vi "03 Channel Tester.vi"() -> ()   [LabVIEW 2009]
uses:
  EquipReferences.ctl
  HEWH Tank Indicator.ctl
  Sensor.ctl
  <vilib>/Instr/_visa.llb/VISA Configure Serial Port (Instr).vi
  <vilib>/Analysis/NI_AALBase.lvlib
panel:
  out "Serial Loopback":cluster{"Com OK":dbl, "Color Box":u32}={"Com OK"=0.0, "Color Box"=8585007}
  in  "RTD Min OK":dbl=30.0
  in  "RTD Max OK":dbl=180.0
  in  "PSI Min OK":dbl=100.0
  in  "PSI Max OK":dbl=400.0
  in  "StDev Thresh":dbl=0.2
  in  "TC Min OK Val":dbl=20.0
  in  "TC Max OK Val":dbl=400.0
  out "Pressures":T1[](array[typedef])=[{"Mean"=0.0, " St Dev."=0.0, "Color Box"=8585007}, {"Mean"=0.0, " St Dev."=0.0, "Color Box"=8585007}, {"Mean"=0.0, " St Dev."=0.0, "Color Box"=8585007}]
  out "Temperatures":T1[](array[typedef])=[{"Mean"=0.0, " St Dev."=0.0, "Color Box"=8585007}, {"Mean"=0.0, " St Dev."=0.0, "Color Box"=8585007}, {"Mean"=0.0, " St Dev."=0.0, "Color Box"=8585007}]
  out "Tc Down":T1={"Mean"=0.0, " St Dev."=0.0, "Color Box"=8585007}
  out "Power":T1={"Mean"=0.0, " St Dev."=0.0, "Color Box"=8585007}
  in  "Panel 3":T1[][](array[typedef])=[[{"Mean"=0.0, " St Dev."=0.0, "Color Box"=8585007}, {"Mean"=0.0, " St Dev."=0.0, "Color Box"=8585007}, {"Mean"=0.0, " St Dev."=0.0, "Color Box"=8585007}, {"Mean"=0.0, " St Dev."=0.0, "Color Box"=8585007}, {"Mean"=0.0, " St Dev."=0.0, "Color Box"=8585007}, {"Mean"=0.0, " St Dev."=0.0, "Color Box"=8585007}], [{"Mean"=0.0, " St Dev."=0.0, "Color Box"=8585007}, {"Mean"=0.0, " St Dev."=0.0, "Color Box"=8585007}, {"Mean"=0.0, " St Dev."=0.0, "Color Box"=8585007}, {"Mean"=0.0, " St Dev."=0.0, "Color Box"=8585007}, {"Mean"=0.0, " St Dev."=0.0, "Color Box"=8585007}, {"Mean"=0.0, " St Dev."=0.0, "Color Box"=8585007}], [{"Mean"=0.0, " St Dev."=0.0, "Color Box"=8585007}, {"Mean"=0.0, " St Dev."=0.0, "Color Box"=8585007}, {"Mean"=0.0, " St Dev."=0.0, "Color Box"=8585007}, {"Mean"=0.0, " St Dev."=0.0, "Color Box"=8585007}, {"Mean"=0.0, " St Dev."=0.0, "Color Box"=8585007}, {"Mean"=0.0, " St Dev."=0.0, "Color Box"=8585007}]]
  in  "Panel 2":T1[][](array[typedef])=[[{"Mean"=0.0, " St Dev."=0.0, "Color Box"=8585007}, {"Mean"=0.0, " St Dev."=0.0, "Color Box"=8585007}, {"Mean"=0.0, " St Dev."=0.0, "Color Box"=8585007}, {"Mean"=0.0, " St Dev."=0.0, "Color Box"=8585007}, {"Mean"=0.0, " St Dev."=0.0, "Color Box"=8585007}, {"Mean"=0.0, " St Dev."=0.0, "Color Box"=8585007}], [{"Mean"=0.0, " St Dev."=0.0, "Color Box"=8585007}, {"Mean"=0.0, " St Dev."=0.0, "Color Box"=8585007}, {"Mean"=0.0, " St Dev."=0.0, "Color Box"=8585007}, {"Mean"=0.0, " St Dev."=0.0, "Color Box"=8585007}, {"Mean"=0.0, " St Dev."=0.0, "Color Box"=8585007}, {"Mean"=0.0, " St Dev."=0.0, "Color Box"=8585007}], [{"Mean"=0.0, " St Dev."=0.0, "Color Box"=8585007}, {"Mean"=0.0, " St Dev."=0.0, "Color Box"=8585007}, {"Mean"=0.0, " St Dev."=0.0, "Color Box"=8585007}, {"Mean"=0.0, " St Dev."=0.0, "Color Box"=8585007}, {"Mean"=0.0, " St Dev."=0.0, "Color Box"=8585007}, {"Mean"=0.0, " St Dev."=0.0, "Color Box"=8585007}]]
  in  "Panel 1":T1[][](array[typedef])=[[{"Mean"=0.0, " St Dev."=0.0, "Color Box"=8585007}, {"Mean"=0.0, " St Dev."=0.0, "Color Box"=8585007}, {"Mean"=0.0, " St Dev."=0.0, "Color Box"=8585007}, {"Mean"=0.0, " St Dev."=0.0, "Color Box"=8585007}, {"Mean"=0.0, " St Dev."=0.0, "Color Box"=8585007}, {"Mean"=0.0, " St Dev."=0.0, "Color Box"=8585007}], [{"Mean"=0.0, " St Dev."=0.0, "Color Box"=8585007}, {"Mean"=0.0, " St Dev."=0.0, "Color Box"=8585007}, {"Mean"=0.0, " St Dev."=0.0, "Color Box"=8585007}, {"Mean"=0.0, " St Dev."=0.0, "Color Box"=8585007}, {"Mean"=0.0, " St Dev."=0.0, "Color Box"=8585007}, {"Mean"=0.0, " St Dev."=0.0, "Color Box"=8585007}], [{"Mean"=0.0, " St Dev."=0.0, "Color Box"=8585007}, {"Mean"=0.0, " St Dev."=0.0, "Color Box"=8585007}, {"Mean"=0.0, " St Dev."=0.0, "Color Box"=8585007}, {"Mean"=0.0, " St Dev."=0.0, "Color Box"=8585007}, {"Mean"=0.0, " St Dev."=0.0, "Color Box"=8585007}, {"Mean"=0.0, " St Dev."=0.0, "Color Box"=8585007}]]
  out "Data Sample":i32
  out "serial error out":errorcluster
  out "Com Port Timeout Value":u32
  out "Local Tank Display":T2 {"TC6" format="%.2g"; "TIN" format="%.2g"; "TOUT" format="%.2g"; "Mean" format="%.2f"; "Std Dev" format="%.2f"; "TC5" format="%.2g"; "TC4" format="%.2g"; "TC3" format="%.2g"; "TC2" format="%.2g"; "TC1" format="%.2g"}
  in  "Num Samples":i32=5
  in  "COM Port":refnum<visa-resource-name>="COM3"
  in  "Semiphore":T3
  in  "error in (no error)":errorcluster
  in  "Equipment":T4={"COM Port"="COM1", "MW100"="MW100", "AG34970"="A-34972A", "Chamber"="WT500"}
  in  "Serial Test":bool
  in  "Test DAQ":bool
  in  "OK":bool
  # "HEWH Pannel Channel Tester"
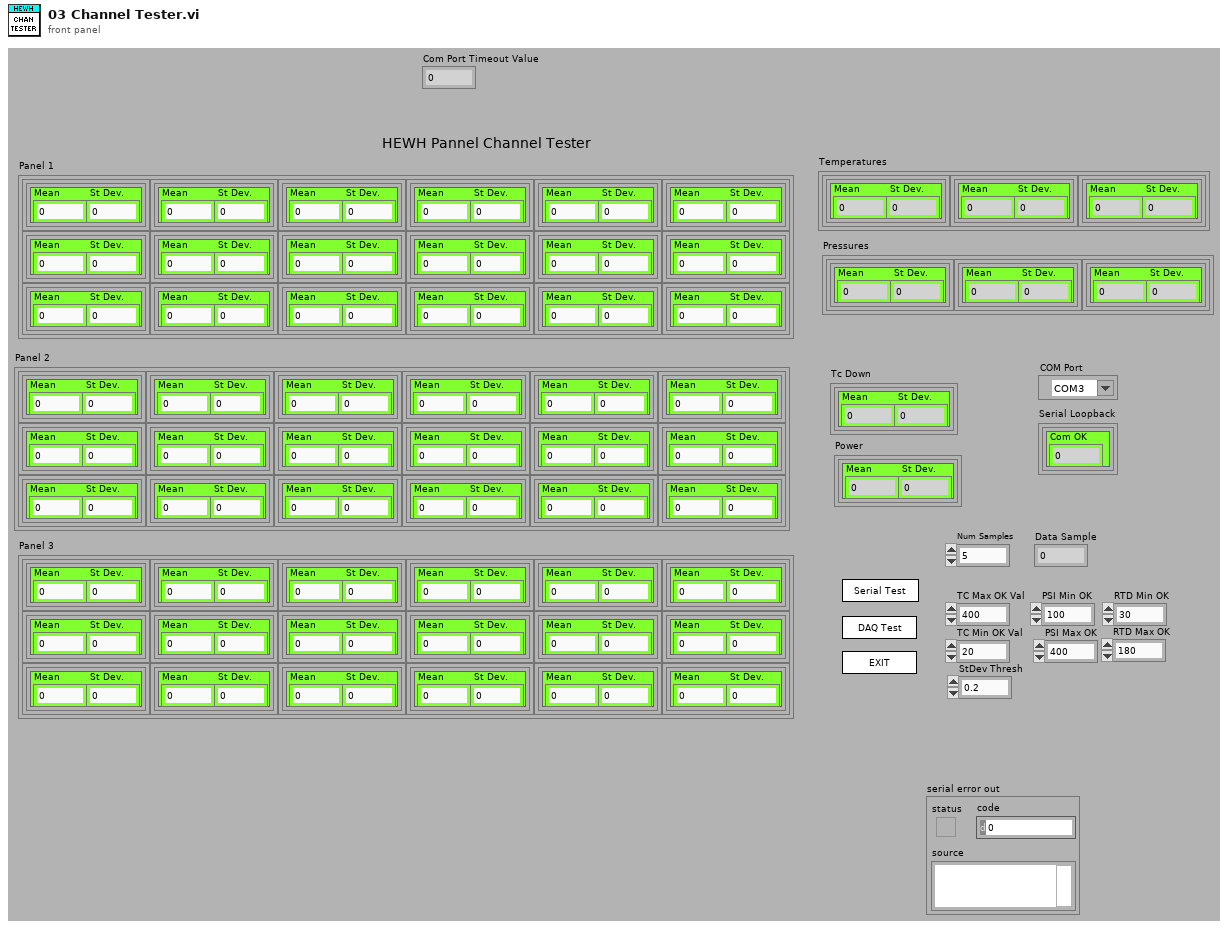
[diagram p1: front panel]
types:
  T1 = typedef "Sensor.ctl" = cluster{"Mean":dbl, " St Dev.":dbl, "Color Box":u32}
  T2 = typedef "HEWH Tank Indicator.ctl" = cluster{"TC1-D":bool, "TC2-D":bool, "TC3-D":bool, "TC4-D":bool, "TC5-D":bool, "RTD_IN":bool, "RTDOUT":bool, "TC1":dbl, "TC2":dbl, "TC3":dbl, "TC4":dbl, "TC5":dbl, "TIN":dbl, "TOUT":dbl, "Std Dev":dbl, "Mean":dbl, "TC6-D":bool, "TC6":dbl}
  T3 = typedef "Semaphore RefNum" = refnum<k1>
  T4 = typedef "EquipReferences.ctl" = cluster{"COM Port":refnum<visa-resource-name>, "MW100":refnum<visa-resource-name>, "AG34970":refnum<visa-resource-name>, "Chamber":refnum<visa-resource-name>}
  T5 = enum32{"invalid app kind", "Development System", "Run Time System", "Student Edition", "Embedded LabVIEW", "Evaluation", "Custom"}
  T6 = enum32{"Invalid", "Standard", "Closed", "Hidden", "Minimized", "Maximized"}
  T7 = cluster{"Core":cluster{"Current VI Reference":refnum<vi>, "Close Panel on Exit?":bool}, "Num Samples":i32, "Equipment Out":T4, "semaphore":T3, "Timeout":u32, "Test Data Array":T1[]}
  T8 = cluster{"Current VI Reference":refnum<vi>, "Close Panel on Exit?":bool}
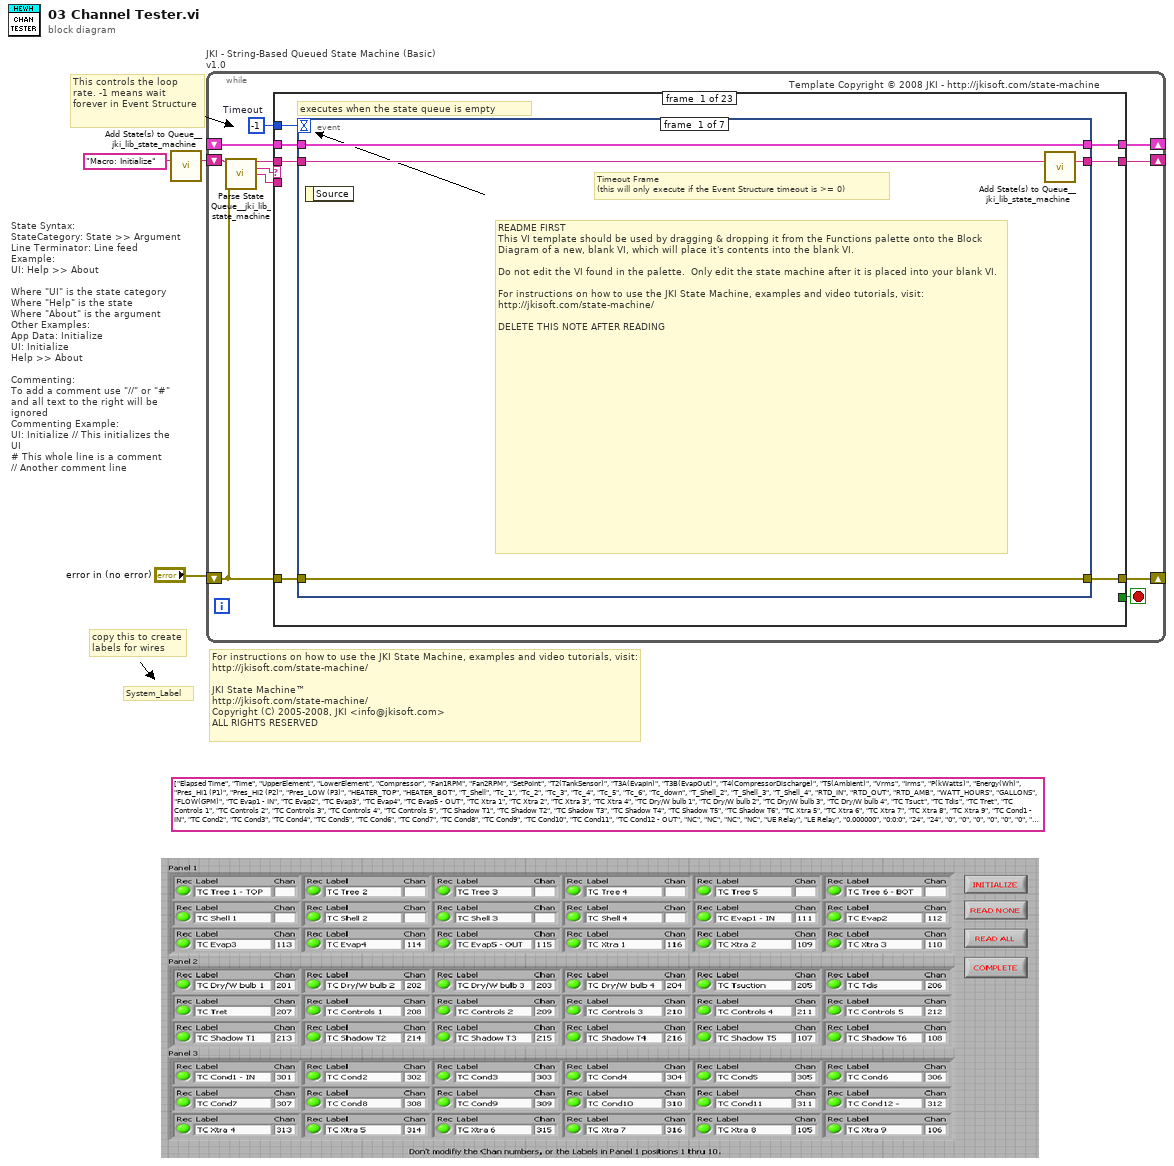
[diagram p0: block diagram]
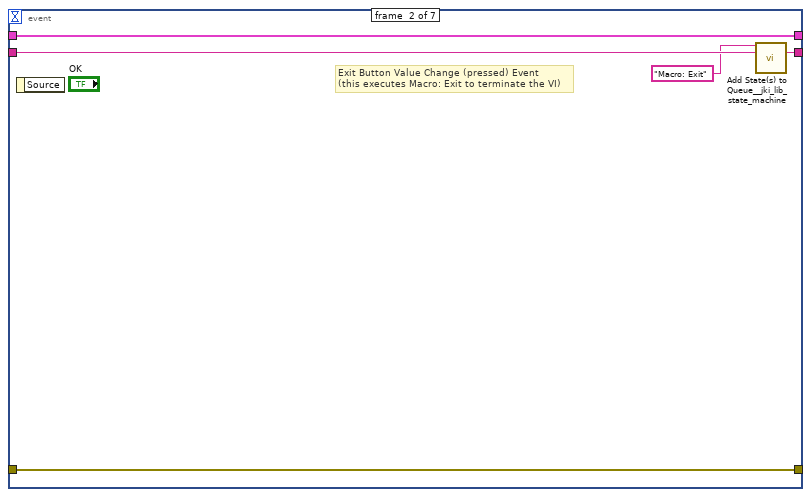
[diagram p2: hidden frame]
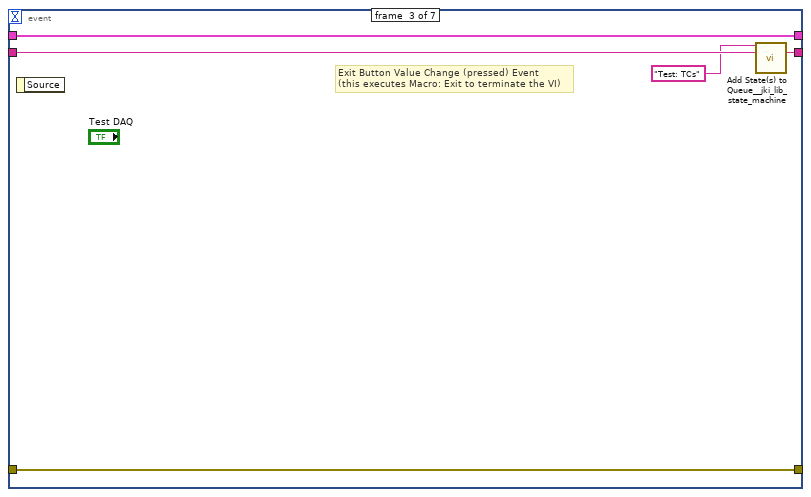
[diagram p3: hidden frame]
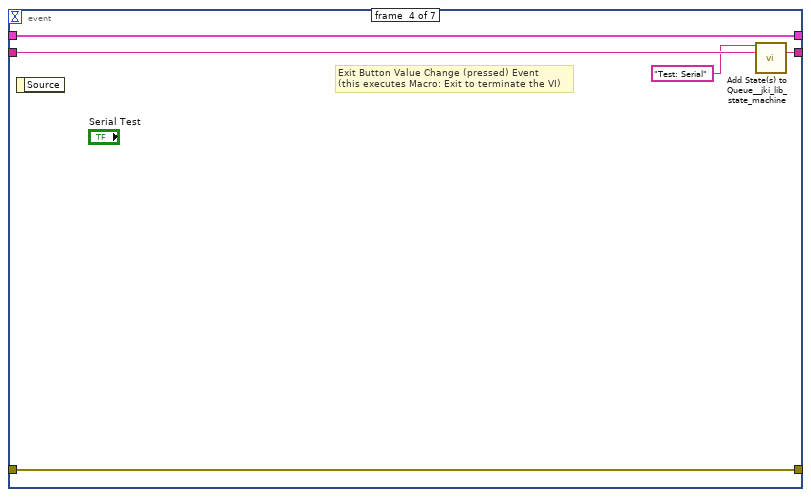
[diagram p4: hidden frame]
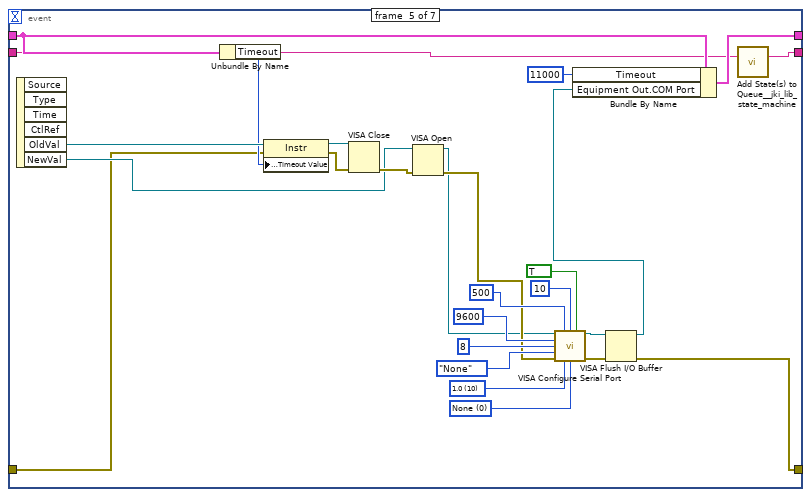
[diagram p5: hidden frame]
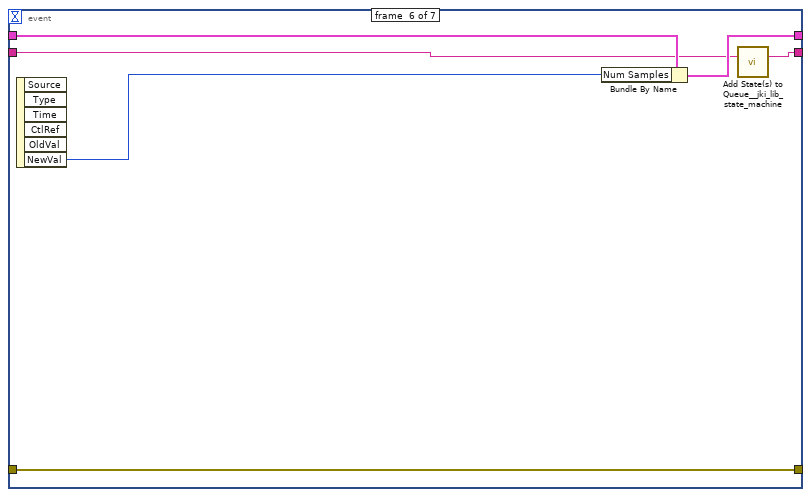
[diagram p6: hidden frame]
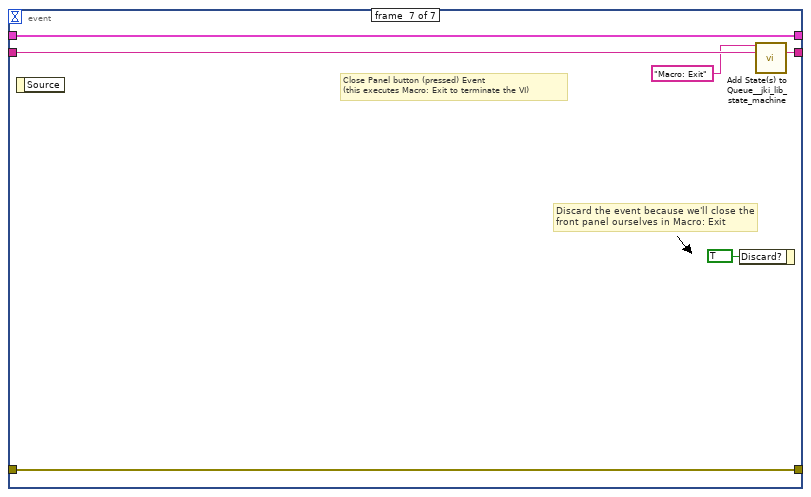
[diagram p7: hidden frame]
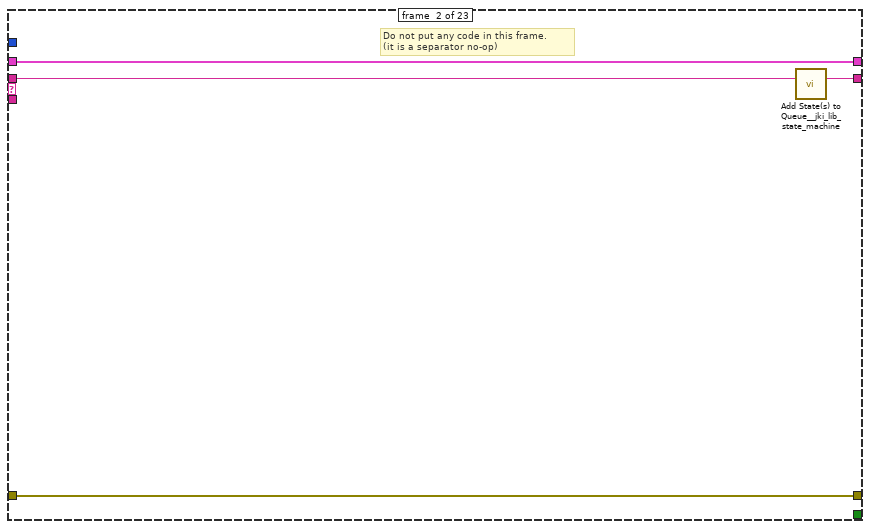
[diagram p8: hidden frame]
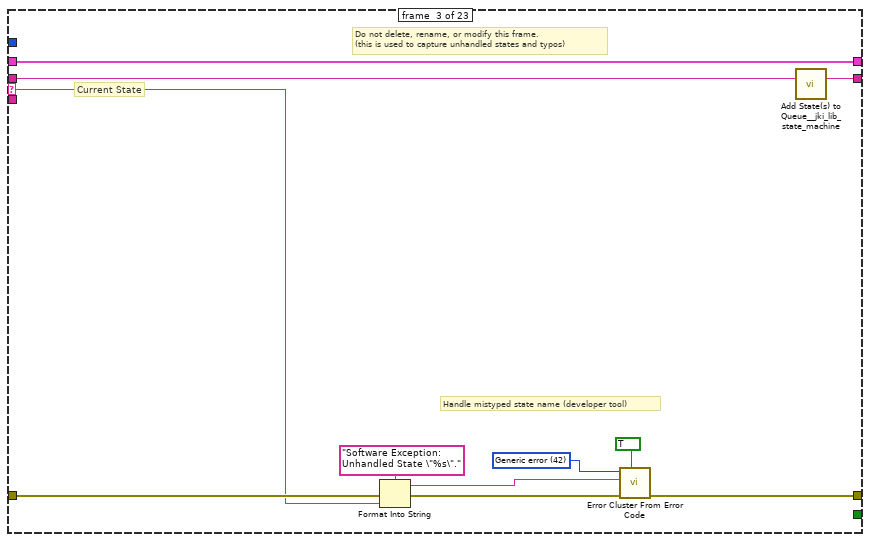
[diagram p9: hidden frame]
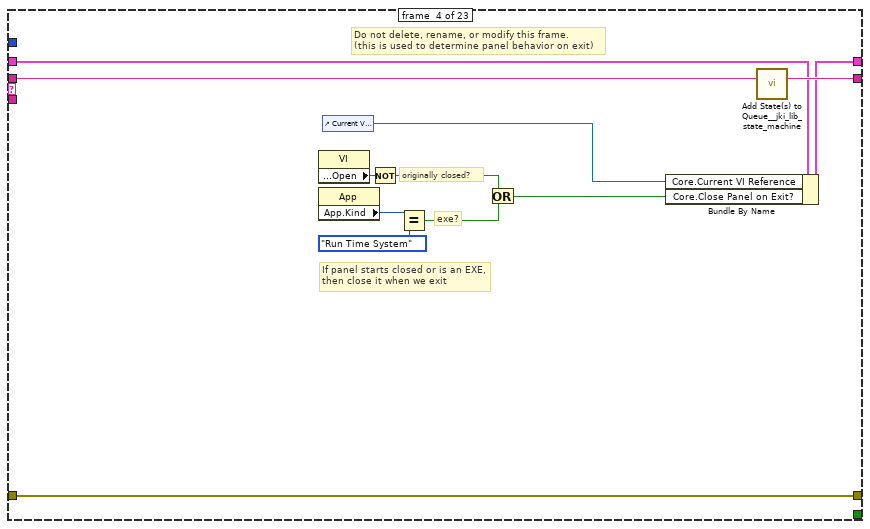
[diagram p10: hidden frame]
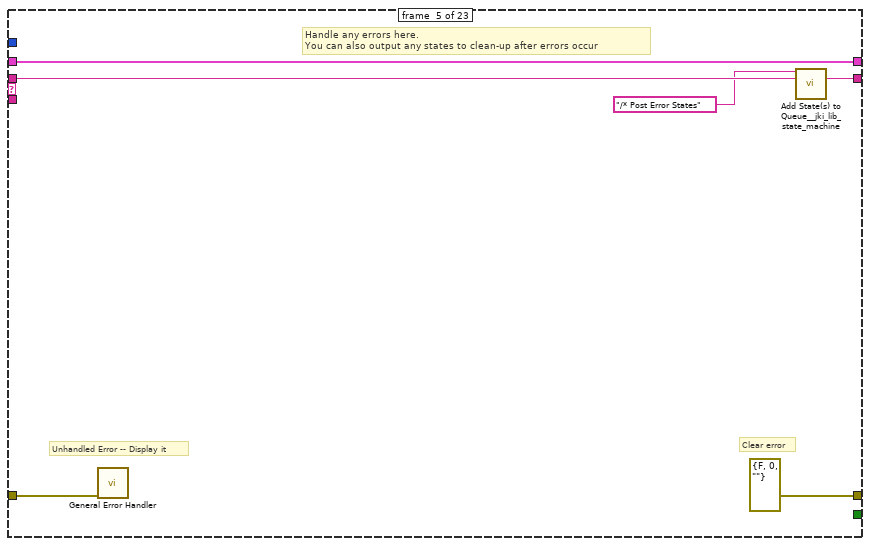
[diagram p11: hidden frame]
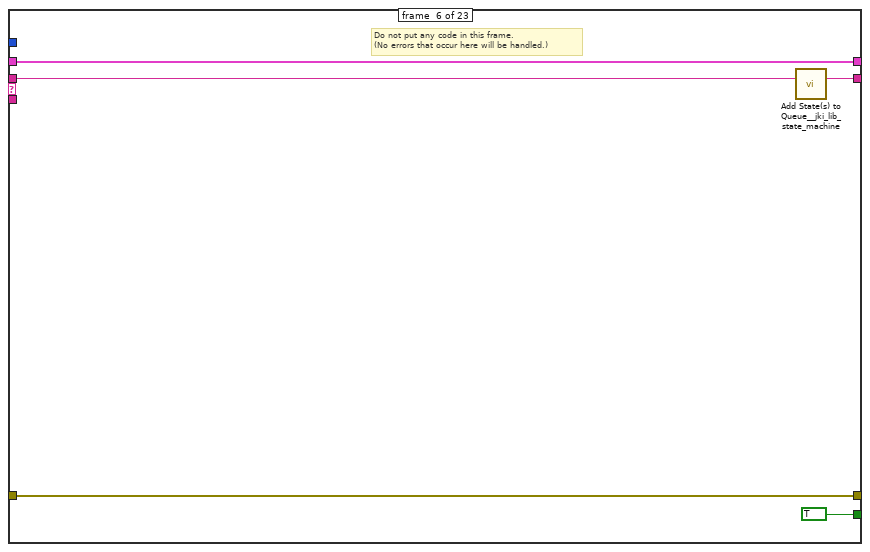
[diagram p12: hidden frame]
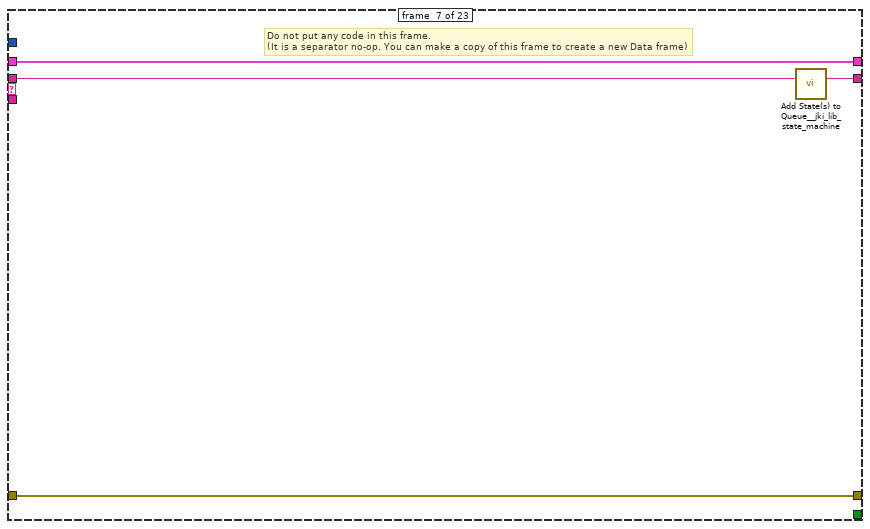
[diagram p13: hidden frame]
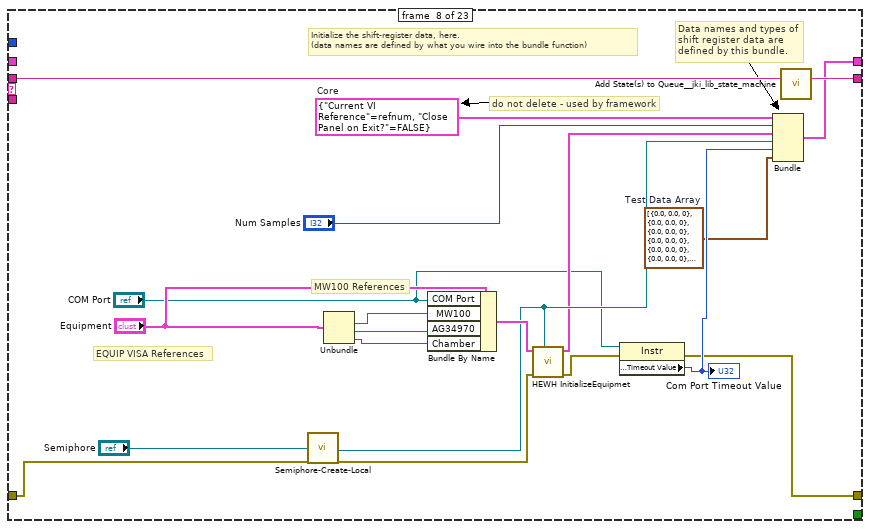
[diagram p14: hidden frame]
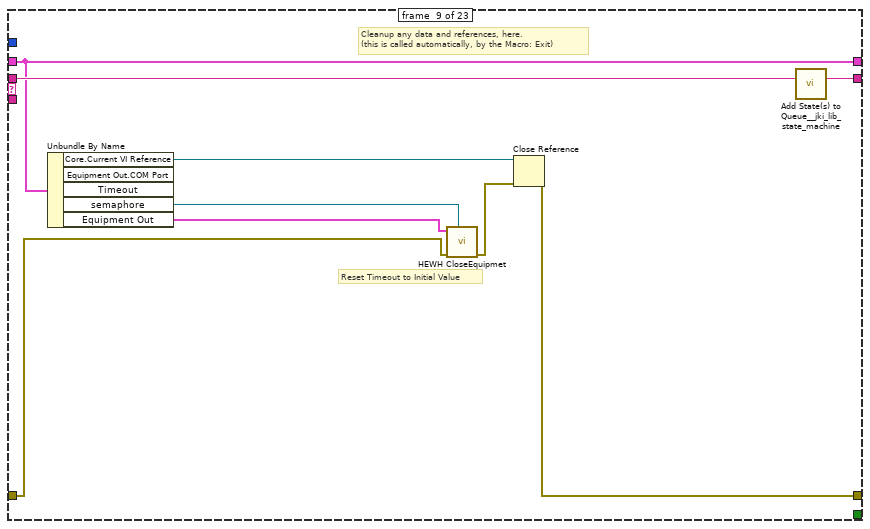
[diagram p15: hidden frame]
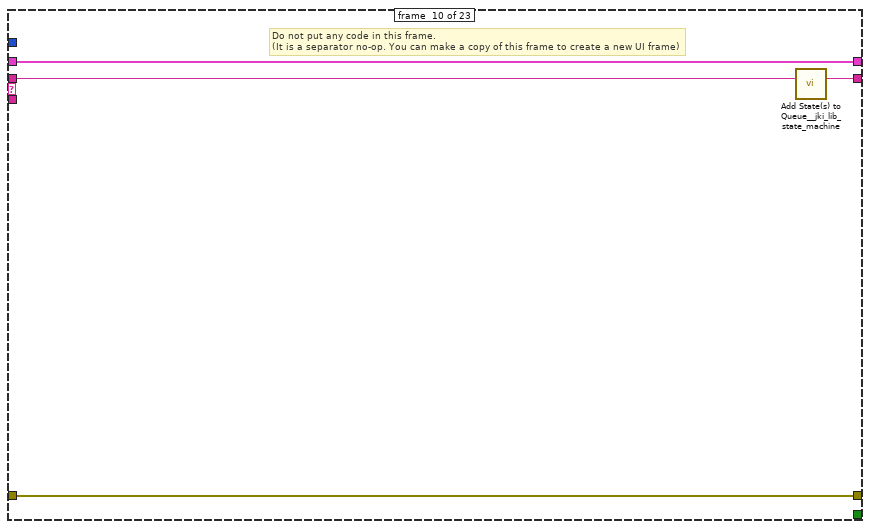
[diagram p16: hidden frame]
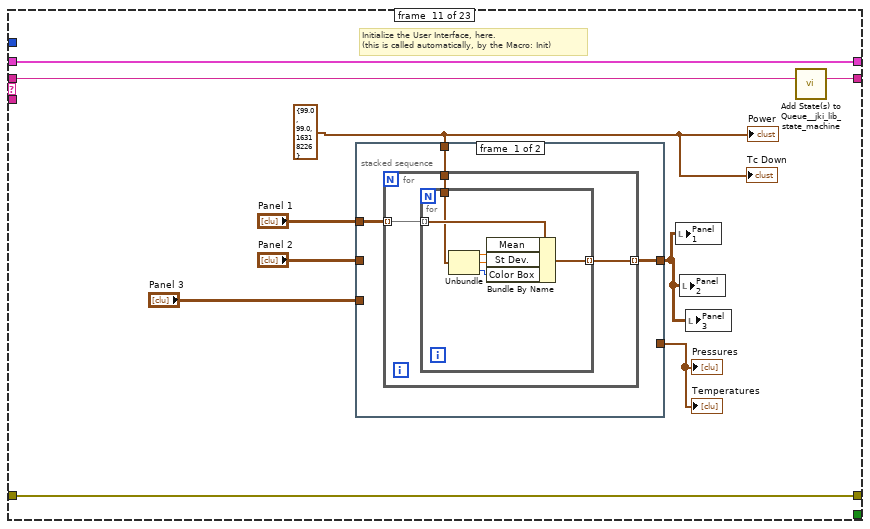
[diagram p17: hidden frame]
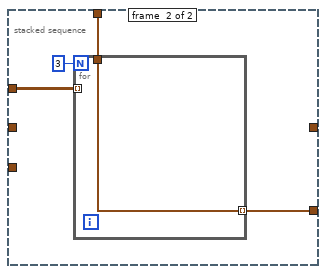
[diagram p18: hidden frame]
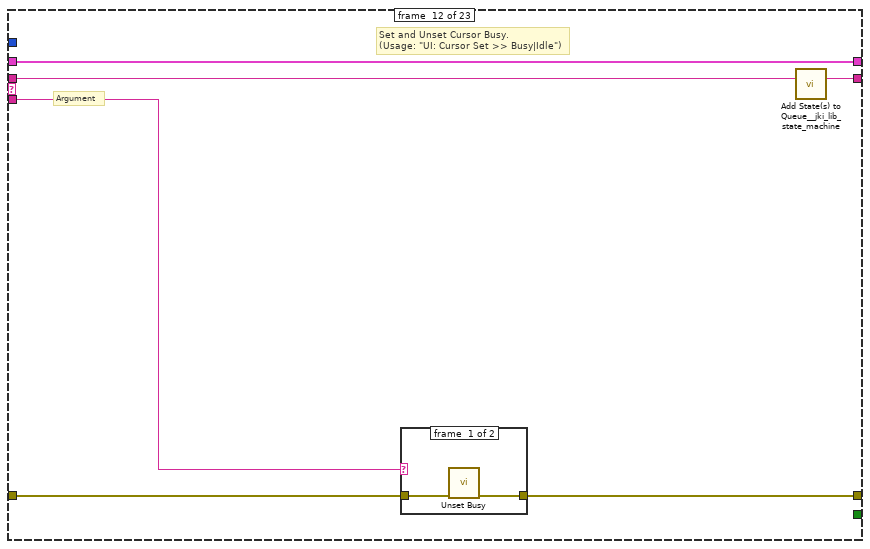
[diagram p19: hidden frame]
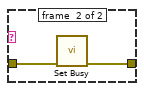
[diagram p20: hidden frame]
diagram:
  (unwired) string[][] [["Elapsed Time", "Time", "UpperElement", "LowerElement", "Compressor", "Fan1RPM", "Fan2RPM", "SetPoint", "T2(TankSensor)", "T3A(EvapIn)", "T3B(EvapOut)", "T4(CompressorDischarge)", "T5(Ambient)", "Vrms", "Irms", "P(kWatts)", "Energy(Wh)", "Pres_HI1 (P1)", "Pres_HI2 (P2)", "Pres_LOW (P3)", "HEATER_TOP", "HEATER_BOT", "T_Shell", "Tc_1", "Tc_2", "Tc_3", "Tc_4", "Tc_5", "Tc_6", "Tc_down", "T_Shell_2", "T_Shell_3", "T_Shell_4", "RTD_IN", "RTD_OUT", "RTD_AMB", "WATT_HOURS", "GALLONS", "FLOW(GPM)", "TC Evap1 - IN", "TC Evap2", "TC Evap3", "TC Evap4", "TC Evap5 - OUT", "TC Xtra 1", "TC Xtra 2", "TC Xtra 3", "TC Xtra 4", "TC Dry/W bulb 1", "TC Dry/W bulb 2", "TC Dry/W bulb 3", "TC Dry/W bulb 4", "TC Tsuct", "TC Tdis", "TC Tret", "TC Controls 1", "TC Controls 2", "TC Controls 3", "TC Controls 4", "TC Controls 5", "TC Shadow T1", "TC Shadow T2", "TC Shadow T3", "TC Shadow T4", "TC Shadow T5", "TC Shadow T6", "TC Xtra 5", "TC Xtra 6", "TC Xtra 7", "TC Xtra 8", "TC Xtra 9", "TC Cond1 - IN", "TC Cond2", "TC Cond3", "TC Cond4", "TC Cond5", "TC Cond6", "TC Cond7", "TC Cond8", "TC Cond9", "TC Cond10", "TC Cond11", "TC Cond12 - OUT", "NC", "NC", "NC", "NC", "UE Relay", "LE Relay"], ["0.000000", "0:0:0", "24", "24", "0", "0", "0", "0", "0", "0", "0", "0", "0", "-229.980000", "-0.000013", "0.003000", "0.000000", "68.20", "67.08", "68.20", "1.00", "1.00", "214745087.90", "63.60", "63.80", "63.90", "63.70", "63.60", "63.90", "69.60", "-322.40", "-318.30", "-214738534.30", "-214738534.30", "-214738534.30", "52.30", "0.00", "0.30", "0.00", "534.04", "-178199999999999999000000000000000000000.00", "55.58", "55.35", "57.06", "55.53", "55.22", "-178199999999999999000000000000000000000.00", "-178199999999999999000000000000000000000.00", "53.73", "54.09", "-178199999999999999000000000000000000000.00", "-178199999999999999000000000000000000000.00", "303.05", "-178199999999999999000000000000000000000.00", "178199999999999999000000000000000000000.00", "-178199999999999999000000000000000000000.00", "460.73", "626.99", "-178199999999999999000000000000000000000.00", "178199999999999999000000000000000000000.00", "-178199999999999999000000000000000000000.00", "131.37", "178199999999999999000000000000000000000.00", "-178199999999999999000000000000000000000.00", "-178199999999999999000000000000000000000.00", "409.13", "259.86", "-178199999999999999000000000000000000000.00", "178199999999999999000000000000000000000.00", "-178199999999999999000000000000000000000.00", "-57.06", "62.09", "61.89", "61.87", "62.14", "62.63", "178199999999999999000000000000000000000.00", "-178199999999999999000000000000000000000.00", "178199999999999999000000000000000000000.00", "-70.58", "-178199999999999999000000000000000000000.00", "178199999999999999000000000000000000000.00", "-178199999999999999000000000000000000000.00", "393.52", "116.86", "83.34", "59.96", "0", "0"]] ("Output Data")
  # "For instructions on how to use the JKI State Machine, examples and video tutorials, visit:\nhttp://jkisoft.com/state-machine/\n\nJKI State Machine™\nhttp://jkisoft.com/state-machine/\nCopyright (C) 2005-2008, JKI <info@jkisoft.com>\nALL RIGHTS RESERVED"
  # "State Syntax:\nStateCategory: State >> Argument\nLine Terminator: Line feed\nExample:\nUI: Help >> About\n\nWhere \"UI\" is the state category\nWhere \"Help\" is the state\nWhere \"About\" is the argument\nOther Examples:\nApp Data: Initialize\nUI: Initialize\nHelp >> About\n\nCommenting:\nTo add a comment use \"//\" or \"#\" and all text to the right will be ignored\nCommenting Example:\nUI: Initialize // This initializes the UI\n# This whole line is a comment\n// Another comment line"
  # "copy this to create labels for wires"
  # "This controls the loop rate. -1 means wait forever in Event Structure"
  # "System_Label"
  n1 = call <vilib>:"Add State(s) to Queue__jki_lib_state_machine.vi"("State(s) in (\"\")"="Macro: Initialize") -> ("States Out"=w3:string)  [unwired: 14 in]
  n2 = while "JKI - String-Based Queued State Machine (Basic) v1.0" {
    shift-right: [w7] -> _
    shift-left: _ -> [w6]
    shift-right: [w10] -> _
    shift-left: "error in (no error)" -> [w4]
    shift-right: [w9] -> _
    shift-left: w3 -> [w11]
    stop <- w8 stop-if-true
    w5 = -1  # Timeout
    # "Template Copyright © 2008 JKI - http://jkisoft.com/state-machine"
    n3 = call <vilib>:"Parse State Queue__jki_lib_state_machine.vi"("State Queue"=w11, "Error In (no error)"=w4) -> ("Remaining States"=w13:string, "Current State"=w14:string, "Arguments"=w12:string)  [unwired: 11 in]
    n4 = case shown="\"Test: Serial\"" w14 {
      selector: w14 -> [_ _ w83 _ _ _ _ _ _ _ _ _ _ _ _ _ _ _ _ _ _ _ _]
      tunnel: w13 -> [w21 w82 w87 w105 w111 w116 w120 w140 w149 w153 w163 w186 w197 w223 w228 w238 w242 w247 w267 w284 w296 w323 w408]
      tunnel: w12 -> [_ _ _ _ _ _ _ _ _ _ _ w181 w191 _ _ _ _ _ _ _ _ _ _]
      tunnel: w6 -> [w19 w79 w85 w96 w108 w114 w117 _ w145 w150 w161 w184 w193 w220 w225 w235 w239 w245 w265 w281 w289 w320 w405]
      tunnel: [w18 w80 w89 w102 errorcluster {"status"=FALSE, "code"=0, "source"=""} ("error out") w113 w118 w122 w146 w151 w160 w182 w194 w221 w226 w236 w240 w243 w255 w282 w293 w321 w406] -> w10
      tunnel: w4 -> [w17 w80 w88 w102 w107 w113 w118 w127 w141 w151 w160 w183 w195 w221 w226 w236 w240 w243 w255 w282 w294 w321 w406]
      tunnel: [w20 w81 w86 w104 w110 w115 w119 w139 w148 w152 w162 w185 w196 w222 w227 w237 w241 w246 w266 w283 w295 w322 w407] -> w9
      tunnel: [_ _ _ _ _ TRUE _ _ _ _ _ _ _ _ _ _ _ _ _ _ _ _ _] -> w8
      tunnel: [w16 w79 w85 w103 w108 w114 w117 w138 w145 w150 w161 w184 w193 w220 w225 w235 w239 w245 w265 w281 w287 w320 w405] -> w7
      tunnel: w5 -> [w15 _ _ _ _ _ _ _ _ _ _ _ _ _ _ _ _ _ _ _ _ _ _]
      frame #0 {
        # "executes when the state queue is empty"
        n5 = event shown="[5] \"Num Samples\": Value Change" {
          selector: _ -> [_ _ _ _ _ _ _]
          dyn-events: _ -> [_ _ _ _ _ _ _]
          timeout: w15 -> [_ _ _ _ _ _ _]
          tunnel: w21 -> [w25 w30 w35 w40 w45 w70 w78]
          tunnel: [w24 w29 w34 w39 w44 w69 w77] -> w20
          tunnel: w19 -> [w22 w27 w32 w37 w62 w72 w75]
          tunnel: [w23 w28 w33 w38 w42 w68 w76] -> w18
          tunnel: w17 -> [w23 w28 w33 w38 w48 w68 w76]
          tunnel: [w22 w27 w32 w37 w46 w71 w75] -> w16
          event #0 {
            # "README FIRST\nThis VI template should be used by dragging & dropping it from the Functions palette onto the Block Diagram of a new, blank VI, which will place it's contents into the blank VI.\n\nDo not edit the VI found in the palette.  Only edit the state machine after it is placed into your blank VI.\n\nFor instructions on how to use the JKI State Machine, examples and video tutorials, visit:\nhttp://jkisoft.com/state-machine/\n\nDELETE THIS NOTE AFTER READING"
            # "Timeout Frame\n(this will only execute if the Event Structure timeout is >= 0)"
            n6 = event-data() -> ()  [unwired: 1 in, 1 out]
            n7 = call <vilib>:"Add State(s) to Queue__jki_lib_state_machine.vi"("State(s) in (\"\")"=w25) -> ("States Out"=w24:string)  [unwired: 14 in]
          }
          event #1 {
            # "Exit Button Value Change (pressed) Event\n(this executes Macro: Exit to terminate the VI)"
            n8 = event-data() -> ()  [unwired: 1 in, 1 out]
            n9 = call <vilib>:"Add State(s) to Queue__jki_lib_state_machine.vi"("State(s) in Front (\"\")"="Macro: Exit", "State(s) in (\"\")"=w30) -> ("States Out"=w29:string)  [unwired: 13 in]
          }
          event #2 {
            # "Exit Button Value Change (pressed) Event\n(this executes Macro: Exit to terminate the VI)"
            n10 = event-data() -> ()  [unwired: 1 in, 1 out]
            n11 = call <vilib>:"Add State(s) to Queue__jki_lib_state_machine.vi"("State(s) in Front (\"\")"="Test: TCs", "State(s) in (\"\")"=w35) -> ("States Out"=w34:string)  [unwired: 13 in]
          }
          event #3 {
            # "Exit Button Value Change (pressed) Event\n(this executes Macro: Exit to terminate the VI)"
            n12 = event-data() -> ()  [unwired: 1 in, 1 out]
            n13 = call <vilib>:"Add State(s) to Queue__jki_lib_state_machine.vi"("State(s) in Front (\"\")"="Test: Serial", "State(s) in (\"\")"=w40) -> ("States Out"=w39:string)  [unwired: 13 in]
          }
          event #4 {
            w57 = u16 0 items=["None", "XON/XOFF", "RTS/CTS", "XON/XOFF & RTS/CTS", "DTR/DSR", "XON/XOFF & DTR/DSR"] ("flow control (0:none)")
            w56 = u16 10 items=["1.0"=10, "1.5"=15, "2.0"=20] ("stop bits (10: 1 bit)")
            n14 = event-data() -> ("OldVal"=w66:refnum<visa-resource-name>, "NewVal"=w50:refnum<visa-resource-name>)  [unwired: 1 in, 4 out]
            n15 = Unbundle By Name(w62) -> ("Timeout"=w65:u32)
            n16 = property class="Instr"(reference=w66, error in=w48, "General Settings:Timeout Value"=w65) -> (reference out=w63:refnum<visa-resource-name>, error out=w64:errorcluster)
            n17 = VISA Close(VISA resource name=w63, error in (no error)=w64) -> (error out=w51:errorcluster)
            n18 = VISA Open(error in (no error)=w51, VISA resource name=w50) -> (VISA resource name=w47:refnum<visa-resource-name>, error out=w49:errorcluster)  [unwired: 3 in]
            n19 = call-poly "VISA Configure Serial Port"("VISA resource name"=w47, "timeout (10sec)"=u32 500, "termination char\n(0xA = '\\n' = LF)"=u8 10 ("termination char\n(0xA = '\\n' = LF)"), "Enable Termination\nChar (T)"=TRUE ("Enable Termination\nChar (T)"), "baud rate (9600)"=u32 9600, "data bits (8)"=u16 8, "parity (0:none)"=enum16{"None", "Odd", "Even", "Mark", "Space"}."None", "error in (no error)"=w49, "stop bits (10: 1 bit)"=w56, "flow control (0:none)"=w57) -> ("VISA resource name out"=w61:refnum<visa-resource-name>, "error out"=w60:errorcluster)  [unwired: 4 in]
            n20 = VISA Flush I/O Buffer(VISA resource name=w61, error in (no error)=w60) -> (VISA resource name out=w43:refnum<visa-resource-name>, error out=w42:errorcluster)  [unwired: 1 in]
            n21 = Bundle By Name(cluster=w62, "Timeout"=u32 11000, "Equipment Out.COM Port"=w43) -> (w46:T7)
            n22 = call <vilib>:"Add State(s) to Queue__jki_lib_state_machine.vi"("State(s) in (\"\")"=w45) -> ("States Out"=w44:string)  [unwired: 14 in]
          }
          event #5 {
            n23 = event-data() -> ("NewVal"=w67:i32)  [unwired: 1 in, 5 out]
            n24 = Bundle By Name(cluster=w72, "Num Samples"=w67) -> (w71:T7)
            n25 = call <vilib>:"Add State(s) to Queue__jki_lib_state_machine.vi"("State(s) in (\"\")"=w70) -> ("States Out"=w69:string)  [unwired: 14 in]
          }
          event #6 {
            # "Discard the event because we'll close the front panel ourselves in Macro: Exit"
            # "Close Panel button (pressed) Event\n(this executes Macro: Exit to terminate the VI)"
            n26 = event-data() -> ()  [unwired: 1 in, 1 out]
            n27 = event-data("Discard?"=TRUE) -> ()  [unwired: 1 in, 1 out]
            n28 = call <vilib>:"Add State(s) to Queue__jki_lib_state_machine.vi"("State(s) in Front (\"\")"="Macro: Exit", "State(s) in (\"\")"=w78) -> ("States Out"=w77:string)  [unwired: 13 in]
          }
        }
      }
      frame #1 {
        # "Do not put any code in this frame.\n(it is a separator no-op)"
        n29 = call <vilib>:"Add State(s) to Queue__jki_lib_state_machine.vi"("State(s) in (\"\")"=w82) -> ("States Out"=w81:string)  [unwired: 14 in]
      }
      frame #2 {
        w92 = 42 items=["No error", "Argument error", "Memory is full", "Out of zone", "End of file", "File already open", "Generic file I/O error", "File not found", "File permission error", "Disk is full", "Duplicate path", "Too many files open", "System feature not enabled", "Resource file not found", "Cannot add resource", "Resource not found", "Image not found", "Image memory error", "Pen does not exist", "Config type invalid", "Config token not found", "Config parse error", "Config memory error", "Bad external code format", "Bad external code offset", "External code not present", "Null window", "Destroy window error", "Null menu", "Print aborted", "Bad print record", "Print driver error", "Windows error during printing", "Memory error during printing", "Print dialog error", "Generic print error", "Invalid device refnum", "Device not found", "Device parameter error", "Device unit error", "Cannot open device", "Device call aborted", "Generic error", "Cancelled by user", "Object ID too low", "Object ID too high", "Object not in heap", "Unknown heap", "Unknown object (invalid DefProc)", "Unknown object (DefProc not in table)", "Message out of range", "Invalid (null) method", "Unknown message", "Manager call not supported", "Bad address", "Network operation in progress", "Network operation timed out", "Connection is busy", "Network attribute not supported", "Network error", "Address in use", "System out of memory", "Connection aborted", "Connection refused", "Not connected", "Already connected", "Connection closed", "Initialization error (interapplication manager)", "Bad occurrence", "Wait on unbound occurrence handler", "Occurrence queue overflow", "Datalog type conflict", "Unused", "Unrecognized type (interapplication manager)", "Memory corrupt", "Failed to make temporary DLL", "Old CIN version", "Drag socket not found", "Failed to load drop-object", "Failed to register OLE object", "Failed to release OLE object", "Format specifier type mismatch", "Unknown format specifier", "Too few format specifiers", "Too many format specifiers", "Scan failed", "Newer CIN version", "Error converting to variant", "Runtime menu error", "Password tampered", "Variant attribute not found", "Incompatible variant data type", "Event data is not available", "Event Store is not present", "Occurrence is not found", "Event Queue is not created", "Event info is not available", "Refnum passed is NULL", "Error retrieving Class GUID", "Error retrieving CoClass GUID", "Error retrieving TypeLib GUID.", "Bad built application magic bytes.", "Specific driver is different from the specific driver associated with the Logical Name.", "There is no session opened to the class driver.", "Max Error", "MAX - Error with config objects", "MAX - Error loading configuration", "MAX - Group not supported"]
        # "Current State"
        # "Do not delete, rename, or modify this frame.\n(this is used to capture unhandled states and typos)"
        # "Handle mistyped state name (developer tool)"
        n30 = Format Into String(format string="Software Exception: Unhandled State \"%s\"." ("message"), error in=w88, w83) -> (resulting string=w91:string, error out=w90:errorcluster)  [unwired: 1 in]
        n31 = call <vilib>:"Error Cluster From Error Code.vi"("show call chain? (False)"=TRUE, "error in (no error)"=w90, "error message (\"\")"=w91, "error code (0)"=w92) -> ("error out"=w89:errorcluster)  [unwired: 5 in]
        n32 = call <vilib>:"Add State(s) to Queue__jki_lib_state_machine.vi"("State(s) in (\"\")"=w87) -> ("States Out"=w86:string)  [unwired: 14 in]
      }
      frame #3 {
        # "Do not delete, rename, or modify this frame.\n(this is used to determine panel behavior on exit)"
        # "originally closed?"
        # "exe?"
        # "If panel starts closed or is an EXE, then close it when we exit"
        n33 = property class="VI"() -> ("Front Panel.Open"=w101:bool)  [unwired: 2 in, 2 out]
        n34 = property class="App"() -> ("App.Kind"=w100:T5)  [unwired: 2 in, 2 out]
        n35 = control-ref of="Current VI Reference"() -> (w94:refnum<vi>)
        n36 = Not(x=w101) -> (.not. x?=w98:bool)
        n37 = Equal?(x=w100, y=T5."Run Time System" ("Application:Kind")) -> (x = y?=w97:bool)
        n38 = Or(x=w98, y=w97) -> (x .or. y?=w95:bool)
        n39 = Bundle By Name(cluster=w96, "Core.Current VI Reference"=w94, "Core.Close Panel on Exit?"=w95) -> (w103:T7)
        n40 = call <vilib>:"Add State(s) to Queue__jki_lib_state_machine.vi"("State(s) in (\"\")"=w105) -> ("States Out"=w104:string)  [unwired: 14 in]
      }
      frame #4 {
        # "Unhandled Error -- Display it"
        # "Handle any errors here.\nYou can also output any states to clean-up after errors occur"
        # "Clear error"
        n41 = call <vilib>:"General Error Handler.vi"("error in (no error)"=w107) -> ()  [unwired: 10 in, 5 out]
        n42 = call <vilib>:"Add State(s) to Queue__jki_lib_state_machine.vi"("State(s) in Front (\"\")"="/* Post Error States", "State(s) in (\"\")"=w111) -> ("States Out"=w110:string)  [unwired: 13 in]
      }
      frame #5 {
        # "Do not put any code in this frame.\n(No errors that occur here will be handled.)"
        n43 = call <vilib>:"Add State(s) to Queue__jki_lib_state_machine.vi"("State(s) in (\"\")"=w116) -> ("States Out"=w115:string)  [unwired: 14 in]
      }
      frame #6 {
        # "Do not put any code in this frame.\n(It is a separator no-op. You can make a copy of this frame to create a new Data frame)"
        n44 = call <vilib>:"Add State(s) to Queue__jki_lib_state_machine.vi"("State(s) in (\"\")"=w120) -> ("States Out"=w119:string)  [unwired: 14 in]
      }
      frame #7 {
        w121 = T1[] [{"Mean"=0.0, " St Dev."=0.0, "Color Box"=0}, {"Mean"=0.0, " St Dev."=0.0, "Color Box"=0}, {"Mean"=0.0, " St Dev."=0.0, "Color Box"=0}, {"Mean"=0.0, " St Dev."=0.0, "Color Box"=0}, {"Mean"=0.0, " St Dev."=0.0, "Color Box"=0}, {"Mean"=0.0, " St Dev."=0.0, "Color Box"=0}, {"Mean"=0.0, " St Dev."=0.0, "Color Box"=0}, {"Mean"=0.0, " St Dev."=0.0, "Color Box"=0}, {"Mean"=0.0, " St Dev."=0.0, "Color Box"=0}, {"Mean"=0.0, " St Dev."=0.0, "Color Box"=0}, {"Mean"=0.0, " St Dev."=0.0, "Color Box"=0}, {"Mean"=0.0, " St Dev."=0.0, "Color Box"=0}, {"Mean"=0.0, " St Dev."=0.0, "Color Box"=0}, {"Mean"=0.0, " St Dev."=0.0, "Color Box"=0}, {"Mean"=0.0, " St Dev."=0.0, "Color Box"=0}, {"Mean"=0.0, " St Dev."=0.0, "Color Box"=0}, {"Mean"=0.0, " St Dev."=0.0, "Color Box"=0}, {"Mean"=0.0, " St Dev."=0.0, "Color Box"=0}, {"Mean"=0.0, " St Dev."=0.0, "Color Box"=0}, {"Mean"=0.0, " St Dev."=0.0, "Color Box"=0}, {"Mean"=0.0, " St Dev."=0.0, "Color Box"=0}, {"Mean"=0.0, " St Dev."=0.0, "Color Box"=0}, {"Mean"=0.0, " St Dev."=0.0, "Color Box"=0}, {"Mean"=0.0, " St Dev."=0.0, "Color Box"=0}, {"Mean"=0.0, " St Dev."=0.0, "Color Box"=0}, {"Mean"=0.0, " St Dev."=0.0, "Color Box"=0}, {"Mean"=0.0, " St Dev."=0.0, "Color Box"=0}, {"Mean"=0.0, " St Dev."=0.0, "Color Box"=0}, {"Mean"=0.0, " St Dev."=0.0, "Color Box"=0}, {"Mean"=0.0, " St Dev."=0.0, "Color Box"=0}, {"Mean"=0.0, " St Dev."=0.0, "Color Box"=0}, {"Mean"=0.0, " St Dev."=0.0, "Color Box"=0}, {"Mean"=0.0, " St Dev."=0.0, "Color Box"=0}, {"Mean"=0.0, " St Dev."=0.0, "Color Box"=0}, {"Mean"=0.0, " St Dev."=0.0, "Color Box"=0}, {"Mean"=0.0, " St Dev."=0.0, "Color Box"=0}, {"Mean"=0.0, " St Dev."=0.0, "Color Box"=0}, {"Mean"=0.0, " St Dev."=0.0, "Color Box"=0}, {"Mean"=0.0, " St Dev."=0.0, "Color Box"=0}, {"Mean"=0.0, " St Dev."=0.0, "Color Box"=0}, {"Mean"=0.0, " St Dev."=0.0, "Color Box"=0}, {"Mean"=0.0, " St Dev."=0.0, "Color Box"=0}, {"Mean"=0.0, " St Dev."=0.0, "Color Box"=0}, {"Mean"=0.0, " St Dev."=0.0, "Color Box"=0}, {"Mean"=0.0, " St Dev."=0.0, "Color Box"=0}, {"Mean"=0.0, " St Dev."=0.0, "Color Box"=0}, {"Mean"=0.0, " St Dev."=0.0, "Color Box"=0}, {"Mean"=0.0, " St Dev."=0.0, "Color Box"=0}, {"Mean"=0.0, " St Dev."=0.0, "Color Box"=0}, {"Mean"=0.0, " St Dev."=0.0, "Color Box"=0}, {"Mean"=0.0, " St Dev."=0.0, "Color Box"=0}, {"Mean"=0.0, " St Dev."=0.0, "Color Box"=0}, {"Mean"=0.0, " St Dev."=0.0, "Color Box"=0}, {"Mean"=0.0, " St Dev."=0.0, "Color Box"=0}, {"Mean"=0.0, " St Dev."=0.0, "Color Box"=0}, {"Mean"=0.0, " St Dev."=0.0, "Color Box"=0}, {"Mean"=0.0, " St Dev."=0.0, "Color Box"=0}, {"Mean"=0.0, " St Dev."=0.0, "Color Box"=0}, {"Mean"=0.0, " St Dev."=0.0, "Color Box"=0}, {"Mean"=0.0, " St Dev."=0.0, "Color Box"=0}, {"Mean"=0.0, " St Dev."=0.0, "Color Box"=0}, {"Mean"=0.0, " St Dev."=0.0, "Color Box"=0}, {"Mean"=0.0, " St Dev."=0.0, "Color Box"=0}, {"Mean"=0.0, " St Dev."=0.0, "Color Box"=0}, {"Mean"=0.0, " St Dev."=0.0, "Color Box"=0}, {"Mean"=0.0, " St Dev."=0.0, "Color Box"=0}, {"Mean"=0.0, " St Dev."=0.0, "Color Box"=0}, {"Mean"=0.0, " St Dev."=0.0, "Color Box"=0}, {"Mean"=0.0, " St Dev."=0.0, "Color Box"=0}, {"Mean"=0.0, " St Dev."=0.0, "Color Box"=0}, {"Mean"=0.0, " St Dev."=0.0, "Color Box"=0}, {"Mean"=0.0, " St Dev."=0.0, "Color Box"=0}, {"Mean"=0.0, " St Dev."=0.0, "Color Box"=0}, {"Mean"=0.0, " St Dev."=0.0, "Color Box"=0}, {"Mean"=0.0, " St Dev."=0.0, "Color Box"=0}, {"Mean"=0.0, " St Dev."=0.0, "Color Box"=0}, {"Mean"=0.0, " St Dev."=0.0, "Color Box"=0}, {"Mean"=0.0, " St Dev."=0.0, "Color Box"=0}, {"Mean"=0.0, " St Dev."=0.0, "Color Box"=0}, {"Mean"=0.0, " St Dev."=0.0, "Color Box"=0}, {"Mean"=0.0, " St Dev."=0.0, "Color Box"=0}, {"Mean"=0.0, " St Dev."=0.0, "Color Box"=0}, {"Mean"=0.0, " St Dev."=0.0, "Color Box"=0}, {"Mean"=0.0, " St Dev."=0.0, "Color Box"=0}, {"Mean"=0.0, " St Dev."=0.0, "Color Box"=0}, {"Mean"=0.0, " St Dev."=0.0, "Color Box"=0}, {"Mean"=0.0, " St Dev."=0.0, "Color Box"=0}, {"Mean"=0.0, " St Dev."=0.0, "Color Box"=0}, {"Mean"=0.0, " St Dev."=0.0, "Color Box"=0}, {"Mean"=0.0, " St Dev."=0.0, "Color Box"=0}, {"Mean"=0.0, " St Dev."=0.0, "Color Box"=0}, {"Mean"=0.0, " St Dev."=0.0, "Color Box"=0}, {"Mean"=0.0, " St Dev."=0.0, "Color Box"=0}, {"Mean"=0.0, " St Dev."=0.0, "Color Box"=0}, {"Mean"=0.0, " St Dev."=0.0, "Color Box"=0}, {"Mean"=0.0, " St Dev."=0.0, "Color Box"=0}, {"Mean"=0.0, " St Dev."=0.0, "Color Box"=0}, {"Mean"=0.0, " St Dev."=0.0, "Color Box"=0}, {"Mean"=0.0, " St Dev."=0.0, "Color Box"=0}, {"Mean"=0.0, " St Dev."=0.0, "Color Box"=0}, {"Mean"=0.0, " St Dev."=0.0, "Color Box"=0}, {"Mean"=0.0, " St Dev."=0.0, "Color Box"=0}, {"Mean"=0.0, " St Dev."=0.0, "Color Box"=0}, {"Mean"=0.0, " St Dev."=0.0, "Color Box"=0}, {"Mean"=0.0, " St Dev."=0.0, "Color Box"=0}, {"Mean"=0.0, " St Dev."=0.0, "Color Box"=0}, {"Mean"=0.0, " St Dev."=0.0, "Color Box"=0}, {"Mean"=0.0, " St Dev."=0.0, "Color Box"=0}, {"Mean"=0.0, " St Dev."=0.0, "Color Box"=0}, {"Mean"=0.0, " St Dev."=0.0, "Color Box"=0}, {"Mean"=0.0, " St Dev."=0.0, "Color Box"=0}, {"Mean"=0.0, " St Dev."=0.0, "Color Box"=0}, {"Mean"=0.0, " St Dev."=0.0, "Color Box"=0}, {"Mean"=0.0, " St Dev."=0.0, "Color Box"=0}, {"Mean"=0.0, " St Dev."=0.0, "Color Box"=0}, {"Mean"=0.0, " St Dev."=0.0, "Color Box"=0}, {"Mean"=0.0, " St Dev."=0.0, "Color Box"=0}, {"Mean"=0.0, " St Dev."=0.0, "Color Box"=0}, {"Mean"=0.0, " St Dev."=0.0, "Color Box"=0}, {"Mean"=0.0, " St Dev."=0.0, "Color Box"=0}, {"Mean"=0.0, " St Dev."=0.0, "Color Box"=0}, {"Mean"=0.0, " St Dev."=0.0, "Color Box"=0}, {"Mean"=0.0, " St Dev."=0.0, "Color Box"=0}, {"Mean"=0.0, " St Dev."=0.0, "Color Box"=0}, {"Mean"=0.0, " St Dev."=0.0, "Color Box"=0}, {"Mean"=0.0, " St Dev."=0.0, "Color Box"=0}, {"Mean"=0.0, " St Dev."=0.0, "Color Box"=0}, {"Mean"=0.0, " St Dev."=0.0, "Color Box"=0}, {"Mean"=0.0, " St Dev."=0.0, "Color Box"=0}, {"Mean"=0.0, " St Dev."=0.0, "Color Box"=0}, {"Mean"=0.0, " St Dev."=0.0, "Color Box"=0}, {"Mean"=0.0, " St Dev."=0.0, "Color Box"=0}, {"Mean"=0.0, " St Dev."=0.0, "Color Box"=0}, {"Mean"=0.0, " St Dev."=0.0, "Color Box"=0}, {"Mean"=0.0, " St Dev."=0.0, "Color Box"=0}, {"Mean"=0.0, " St Dev."=0.0, "Color Box"=0}, {"Mean"=0.0, " St Dev."=0.0, "Color Box"=0}, {"Mean"=0.0, " St Dev."=0.0, "Color Box"=0}, {"Mean"=0.0, " St Dev."=0.0, "Color Box"=0}, {"Mean"=0.0, " St Dev."=0.0, "Color Box"=0}, {"Mean"=0.0, " St Dev."=0.0, "Color Box"=0}, {"Mean"=0.0, " St Dev."=0.0, "Color Box"=0}, {"Mean"=0.0, " St Dev."=0.0, "Color Box"=0}, {"Mean"=0.0, " St Dev."=0.0, "Color Box"=0}, {"Mean"=0.0, " St Dev."=0.0, "Color Box"=0}, {"Mean"=0.0, " St Dev."=0.0, "Color Box"=0}, {"Mean"=0.0, " St Dev."=0.0, "Color Box"=0}, {"Mean"=0.0, " St Dev."=0.0, "Color Box"=0}, {"Mean"=0.0, " St Dev."=0.0, "Color Box"=0}, {"Mean"=0.0, " St Dev."=0.0, "Color Box"=0}, {"Mean"=0.0, " St Dev."=0.0, "Color Box"=0}, {"Mean"=0.0, " St Dev."=0.0, "Color Box"=0}, {"Mean"=0.0, " St Dev."=0.0, "Color Box"=0}, {"Mean"=0.0, " St Dev."=0.0, "Color Box"=0}, {"Mean"=0.0, " St Dev."=0.0, "Color Box"=0}, {"Mean"=0.0, " St Dev."=0.0, "Color Box"=0}, {"Mean"=0.0, " St Dev."=0.0, "Color Box"=0}, {"Mean"=0.0, " St Dev."=0.0, "Color Box"=0}, {"Mean"=0.0, " St Dev."=0.0, "Color Box"=0}, {"Mean"=0.0, " St Dev."=0.0, "Color Box"=0}, {"Mean"=0.0, " St Dev."=0.0, "Color Box"=0}, {"Mean"=0.0, " St Dev."=0.0, "Color Box"=0}, {"Mean"=0.0, " St Dev."=0.0, "Color Box"=0}, {"Mean"=0.0, " St Dev."=0.0, "Color Box"=0}, {"Mean"=0.0, " St Dev."=0.0, "Color Box"=0}, {"Mean"=0.0, " St Dev."=0.0, "Color Box"=0}, {"Mean"=0.0, " St Dev."=0.0, "Color Box"=0}, {"Mean"=0.0, " St Dev."=0.0, "Color Box"=0}, {"Mean"=0.0, " St Dev."=0.0, "Color Box"=0}, {"Mean"=0.0, " St Dev."=0.0, "Color Box"=0}, {"Mean"=0.0, " St Dev."=0.0, "Color Box"=0}, {"Mean"=0.0, " St Dev."=0.0, "Color Box"=0}, {"Mean"=0.0, " St Dev."=0.0, "Color Box"=0}, {"Mean"=0.0, " St Dev."=0.0, "Color Box"=0}, {"Mean"=0.0, " St Dev."=0.0, "Color Box"=0}, {"Mean"=0.0, " St Dev."=0.0, "Color Box"=0}, {"Mean"=0.0, " St Dev."=0.0, "Color Box"=0}, {"Mean"=0.0, " St Dev."=0.0, "Color Box"=0}, {"Mean"=0.0, " St Dev."=0.0, "Color Box"=0}, {"Mean"=0.0, " St Dev."=0.0, "Color Box"=0}, {"Mean"=0.0, " St Dev."=0.0, "Color Box"=0}, {"Mean"=0.0, " St Dev."=0.0, "Color Box"=0}, {"Mean"=0.0, " St Dev."=0.0, "Color Box"=0}, {"Mean"=0.0, " St Dev."=0.0, "Color Box"=0}, {"Mean"=0.0, " St Dev."=0.0, "Color Box"=0}, {"Mean"=0.0, " St Dev."=0.0, "Color Box"=0}, {"Mean"=0.0, " St Dev."=0.0, "Color Box"=0}, {"Mean"=0.0, " St Dev."=0.0, "Color Box"=0}, {"Mean"=0.0, " St Dev."=0.0, "Color Box"=0}, {"Mean"=0.0, " St Dev."=0.0, "Color Box"=0}, {"Mean"=0.0, " St Dev."=0.0, "Color Box"=0}, {"Mean"=0.0, " St Dev."=0.0, "Color Box"=0}, {"Mean"=0.0, " St Dev."=0.0, "Color Box"=0}, {"Mean"=0.0, " St Dev."=0.0, "Color Box"=0}, {"Mean"=0.0, " St Dev."=0.0, "Color Box"=0}, {"Mean"=0.0, " St Dev."=0.0, "Color Box"=0}, {"Mean"=0.0, " St Dev."=0.0, "Color Box"=0}, {"Mean"=0.0, " St Dev."=0.0, "Color Box"=0}, {"Mean"=0.0, " St Dev."=0.0, "Color Box"=0}, {"Mean"=0.0, " St Dev."=0.0, "Color Box"=0}, {"Mean"=0.0, " St Dev."=0.0, "Color Box"=0}, {"Mean"=0.0, " St Dev."=0.0, "Color Box"=0}, {"Mean"=0.0, " St Dev."=0.0, "Color Box"=0}, {"Mean"=0.0, " St Dev."=0.0, "Color Box"=0}, {"Mean"=0.0, " St Dev."=0.0, "Color Box"=0}, {"Mean"=0.0, " St Dev."=0.0, "Color Box"=0}, {"Mean"=0.0, " St Dev."=0.0, "Color Box"=0}, {"Mean"=0.0, " St Dev."=0.0, "Color Box"=0}, {"Mean"=0.0, " St Dev."=0.0, "Color Box"=0}, {"Mean"=0.0, " St Dev."=0.0, "Color Box"=0}, {"Mean"=0.0, " St Dev."=0.0, "Color Box"=0}, {"Mean"=0.0, " St Dev."=0.0, "Color Box"=0}, {"Mean"=0.0, " St Dev."=0.0, "Color Box"=0}, {"Mean"=0.0, " St Dev."=0.0, "Color Box"=0}, {"Mean"=0.0, " St Dev."=0.0, "Color Box"=0}, {"Mean"=0.0, " St Dev."=0.0, "Color Box"=0}, {"Mean"=0.0, " St Dev."=0.0, "Color Box"=0}, {"Mean"=0.0, " St Dev."=0.0, "Color Box"=0}, {"Mean"=0.0, " St Dev."=0.0, "Color Box"=0}, {"Mean"=0.0, " St Dev."=0.0, "Color Box"=0}, {"Mean"=0.0, " St Dev."=0.0, "Color Box"=0}, {"Mean"=0.0, " St Dev."=0.0, "Color Box"=0}, {"Mean"=0.0, " St Dev."=0.0, "Color Box"=0}, {"Mean"=0.0, " St Dev."=0.0, "Color Box"=0}, {"Mean"=0.0, " St Dev."=0.0, "Color Box"=0}, {"Mean"=0.0, " St Dev."=0.0, "Color Box"=0}, {"Mean"=0.0, " St Dev."=0.0, "Color Box"=0}, {"Mean"=0.0, " St Dev."=0.0, "Color Box"=0}, {"Mean"=0.0, " St Dev."=0.0, "Color Box"=0}, {"Mean"=0.0, " St Dev."=0.0, "Color Box"=0}, {"Mean"=0.0, " St Dev."=0.0, "Color Box"=0}, {"Mean"=0.0, " St Dev."=0.0, "Color Box"=0}, {"Mean"=0.0, " St Dev."=0.0, "Color Box"=0}, {"Mean"=0.0, " St Dev."=0.0, "Color Box"=0}, {"Mean"=0.0, " St Dev."=0.0, "Color Box"=0}, {"Mean"=0.0, " St Dev."=0.0, "Color Box"=0}, {"Mean"=0.0, " St Dev."=0.0, "Color Box"=0}, {"Mean"=0.0, " St Dev."=0.0, "Color Box"=0}, {"Mean"=0.0, " St Dev."=0.0, "Color Box"=0}, {"Mean"=0.0, " St Dev."=0.0, "Color Box"=0}, {"Mean"=0.0, " St Dev."=0.0, "Color Box"=0}, {"Mean"=0.0, " St Dev."=0.0, "Color Box"=0}, {"Mean"=0.0, " St Dev."=0.0, "Color Box"=0}, {"Mean"=0.0, " St Dev."=0.0, "Color Box"=0}, {"Mean"=0.0, " St Dev."=0.0, "Color Box"=0}, {"Mean"=0.0, " St Dev."=0.0, "Color Box"=0}, {"Mean"=0.0, " St Dev."=0.0, "Color Box"=0}, {"Mean"=0.0, " St Dev."=0.0, "Color Box"=0}, {"Mean"=0.0, " St Dev."=0.0, "Color Box"=0}, {"Mean"=0.0, " St Dev."=0.0, "Color Box"=0}, {"Mean"=0.0, " St Dev."=0.0, "Color Box"=0}, {"Mean"=0.0, " St Dev."=0.0, "Color Box"=0}, {"Mean"=0.0, " St Dev."=0.0, "Color Box"=0}, {"Mean"=0.0, " St Dev."=0.0, "Color Box"=0}, {"Mean"=0.0, " St Dev."=0.0, "Color Box"=0}, {"Mean"=0.0, " St Dev."=0.0, "Color Box"=0}, {"Mean"=0.0, " St Dev."=0.0, "Color Box"=0}, {"Mean"=0.0, " St Dev."=0.0, "Color Box"=0}, {"Mean"=0.0, " St Dev."=0.0, "Color Box"=0}, {"Mean"=0.0, " St Dev."=0.0, "Color Box"=0}, {"Mean"=0.0, " St Dev."=0.0, "Color Box"=0}, {"Mean"=0.0, " St Dev."=0.0, "Color Box"=0}, {"Mean"=0.0, " St Dev."=0.0, "Color Box"=0}, {"Mean"=0.0, " St Dev."=0.0, "Color Box"=0}, {"Mean"=0.0, " St Dev."=0.0, "Color Box"=0}, {"Mean"=0.0, " St Dev."=0.0, "Color Box"=0}, {"Mean"=0.0, " St Dev."=0.0, "Color Box"=0}, {"Mean"=0.0, " St Dev."=0.0, "Color Box"=0}, {"Mean"=0.0, " St Dev."=0.0, "Color Box"=0}, {"Mean"=0.0, " St Dev."=0.0, "Color Box"=0}, {"Mean"=0.0, " St Dev."=0.0, "Color Box"=0}, {"Mean"=0.0, " St Dev."=0.0, "Color Box"=0}, {"Mean"=0.0, " St Dev."=0.0, "Color Box"=0}, {"Mean"=0.0, " St Dev."=0.0, "Color Box"=0}, {"Mean"=0.0, " St Dev."=0.0, "Color Box"=0}, {"Mean"=0.0, " St Dev."=0.0, "Color Box"=0}, {"Mean"=0.0, " St Dev."=0.0, "Color Box"=0}, {"Mean"=0.0, " St Dev."=0.0, "Color Box"=0}, {"Mean"=0.0, " St Dev."=0.0, "Color Box"=0}, {"Mean"=0.0, " St Dev."=0.0, "Color Box"=0}, {"Mean"=0.0, " St Dev."=0.0, "Color Box"=0}, {"Mean"=0.0, " St Dev."=0.0, "Color Box"=0}, {"Mean"=0.0, " St Dev."=0.0, "Color Box"=0}, {"Mean"=0.0, " St Dev."=0.0, "Color Box"=0}, {"Mean"=0.0, " St Dev."=0.0, "Color Box"=0}, {"Mean"=0.0, " St Dev."=0.0, "Color Box"=0}, {"Mean"=0.0, " St Dev."=0.0, "Color Box"=0}, {"Mean"=0.0, " St Dev."=0.0, "Color Box"=0}, {"Mean"=0.0, " St Dev."=0.0, "Color Box"=0}, {"Mean"=0.0, " St Dev."=0.0, "Color Box"=0}, {"Mean"=0.0, " St Dev."=0.0, "Color Box"=0}, {"Mean"=0.0, " St Dev."=0.0, "Color Box"=0}, {"Mean"=0.0, " St Dev."=0.0, "Color Box"=0}, {"Mean"=0.0, " St Dev."=0.0, "Color Box"=0}, {"Mean"=0.0, " St Dev."=0.0, "Color Box"=0}, {"Mean"=0.0, " St Dev."=0.0, "Color Box"=0}, {"Mean"=0.0, " St Dev."=0.0, "Color Box"=0}, {"Mean"=0.0, " St Dev."=0.0, "Color Box"=0}, {"Mean"=0.0, " St Dev."=0.0, "Color Box"=0}, {"Mean"=0.0, " St Dev."=0.0, "Color Box"=0}, {"Mean"=0.0, " St Dev."=0.0, "Color Box"=0}, {"Mean"=0.0, " St Dev."=0.0, "Color Box"=0}, {"Mean"=0.0, " St Dev."=0.0, "Color Box"=0}, {"Mean"=0.0, " St Dev."=0.0, "Color Box"=0}, {"Mean"=0.0, " St Dev."=0.0, "Color Box"=0}, {"Mean"=0.0, " St Dev."=0.0, "Color Box"=0}, {"Mean"=0.0, " St Dev."=0.0, "Color Box"=0}, {"Mean"=0.0, " St Dev."=0.0, "Color Box"=0}, {"Mean"=0.0, " St Dev."=0.0, "Color Box"=0}, {"Mean"=0.0, " St Dev."=0.0, "Color Box"=0}, {"Mean"=0.0, " St Dev."=0.0, "Color Box"=0}, {"Mean"=0.0, " St Dev."=0.0, "Color Box"=0}, {"Mean"=0.0, " St Dev."=0.0, "Color Box"=0}, {"Mean"=0.0, " St Dev."=0.0, "Color Box"=0}, {"Mean"=0.0, " St Dev."=0.0, "Color Box"=0}, {"Mean"=0.0, " St Dev."=0.0, "Color Box"=0}, {"Mean"=0.0, " St Dev."=0.0, "Color Box"=0}, {"Mean"=0.0, " St Dev."=0.0, "Color Box"=0}, {"Mean"=0.0, " St Dev."=0.0, "Color Box"=0}, {"Mean"=0.0, " St Dev."=0.0, "Color Box"=0}, {"Mean"=0.0, " St Dev."=0.0, "Color Box"=0}, {"Mean"=0.0, " St Dev."=0.0, "Color Box"=0}, {"Mean"=0.0, " St Dev."=0.0, "Color Box"=0}, {"Mean"=0.0, " St Dev."=0.0, "Color Box"=0}, {"Mean"=0.0, " St Dev."=0.0, "Color Box"=0}, {"Mean"=0.0, " St Dev."=0.0, "Color Box"=0}, {"Mean"=0.0, " St Dev."=0.0, "Color Box"=0}, {"Mean"=0.0, " St Dev."=0.0, "Color Box"=0}, {"Mean"=0.0, " St Dev."=0.0, "Color Box"=0}, {"Mean"=0.0, " St Dev."=0.0, "Color Box"=0}, {"Mean"=0.0, " St Dev."=0.0, "Color Box"=0}, {"Mean"=0.0, " St Dev."=0.0, "Color Box"=0}, {"Mean"=0.0, " St Dev."=0.0, "Color Box"=0}, {"Mean"=0.0, " St Dev."=0.0, "Color Box"=0}, {"Mean"=0.0, " St Dev."=0.0, "Color Box"=0}, {"Mean"=0.0, " St Dev."=0.0, "Color Box"=0}, {"Mean"=0.0, " St Dev."=0.0, "Color Box"=0}, {"Mean"=0.0, " St Dev."=0.0, "Color Box"=0}, {"Mean"=0.0, " St Dev."=0.0, "Color Box"=0}, {"Mean"=0.0, " St Dev."=0.0, "Color Box"=0}, {"Mean"=0.0, " St Dev."=0.0, "Color Box"=0}, {"Mean"=0.0, " St Dev."=0.0, "Color Box"=0}, {"Mean"=0.0, " St Dev."=0.0, "Color Box"=0}, {"Mean"=0.0, " St Dev."=0.0, "Color Box"=0}, {"Mean"=0.0, " St Dev."=0.0, "Color Box"=0}, {"Mean"=0.0, " St Dev."=0.0, "Color Box"=0}, {"Mean"=0.0, " St Dev."=0.0, "Color Box"=0}, {"Mean"=0.0, " St Dev."=0.0, "Color Box"=0}, {"Mean"=0.0, " St Dev."=0.0, "Color Box"=0}, {"Mean"=0.0, " St Dev."=0.0, "Color Box"=0}, {"Mean"=0.0, " St Dev."=0.0, "Color Box"=0}, {"Mean"=0.0, " St Dev."=0.0, "Color Box"=0}, {"Mean"=0.0, " St Dev."=0.0, "Color Box"=0}, {"Mean"=0.0, " St Dev."=0.0, "Color Box"=0}, {"Mean"=0.0, " St Dev."=0.0, "Color Box"=0}, {"Mean"=0.0, " St Dev."=0.0, "Color Box"=0}, {"Mean"=0.0, " St Dev."=0.0, "Color Box"=0}, {"Mean"=0.0, " St Dev."=0.0, "Color Box"=0}, {"Mean"=0.0, " St Dev."=0.0, "Color Box"=0}, {"Mean"=0.0, " St Dev."=0.0, "Color Box"=0}, {"Mean"=0.0, " St Dev."=0.0, "Color Box"=0}, {"Mean"=0.0, " St Dev."=0.0, "Color Box"=0}, {"Mean"=0.0, " St Dev."=0.0, "Color Box"=0}, {"Mean"=0.0, " St Dev."=0.0, "Color Box"=0}, {"Mean"=0.0, " St Dev."=0.0, "Color Box"=0}, {"Mean"=0.0, " St Dev."=0.0, "Color Box"=0}, {"Mean"=0.0, " St Dev."=0.0, "Color Box"=0}, {"Mean"=0.0, " St Dev."=0.0, "Color Box"=0}, {"Mean"=0.0, " St Dev."=0.0, "Color Box"=0}, {"Mean"=0.0, " St Dev."=0.0, "Color Box"=0}, {"Mean"=0.0, " St Dev."=0.0, "Color Box"=0}, {"Mean"=0.0, " St Dev."=0.0, "Color Box"=0}, {"Mean"=0.0, " St Dev."=0.0, "Color Box"=0}, {"Mean"=0.0, " St Dev."=0.0, "Color Box"=0}, {"Mean"=0.0, " St Dev."=0.0, "Color Box"=0}, {"Mean"=0.0, " St Dev."=0.0, "Color Box"=0}, {"Mean"=0.0, " St Dev."=0.0, "Color Box"=0}, {"Mean"=0.0, " St Dev."=0.0, "Color Box"=0}, {"Mean"=0.0, " St Dev."=0.0, "Color Box"=0}, {"Mean"=0.0, " St Dev."=0.0, "Color Box"=0}, {"Mean"=0.0, " St Dev."=0.0, "Color Box"=0}, {"Mean"=0.0, " St Dev."=0.0, "Color Box"=0}, {"Mean"=0.0, " St Dev."=0.0, "Color Box"=0}, {"Mean"=0.0, " St Dev."=0.0, "Color Box"=0}, {"Mean"=0.0, " St Dev."=0.0, "Color Box"=0}, {"Mean"=0.0, " St Dev."=0.0, "Color Box"=0}, {"Mean"=0.0, " St Dev."=0.0, "Color Box"=0}, {"Mean"=0.0, " St Dev."=0.0, "Color Box"=0}, {"Mean"=0.0, " St Dev."=0.0, "Color Box"=0}, {"Mean"=0.0, " St Dev."=0.0, "Color Box"=0}, {"Mean"=0.0, " St Dev."=0.0, "Color Box"=0}, {"Mean"=0.0, " St Dev."=0.0, "Color Box"=0}, {"Mean"=0.0, " St Dev."=0.0, "Color Box"=0}, {"Mean"=0.0, " St Dev."=0.0, "Color Box"=0}, {"Mean"=0.0, " St Dev."=0.0, "Color Box"=0}, {"Mean"=0.0, " St Dev."=0.0, "Color Box"=0}, {"Mean"=0.0, " St Dev."=0.0, "Color Box"=0}, {"Mean"=0.0, " St Dev."=0.0, "Color Box"=0}, {"Mean"=0.0, " St Dev."=0.0, "Color Box"=0}, {"Mean"=0.0, " St Dev."=0.0, "Color Box"=0}, {"Mean"=0.0, " St Dev."=0.0, "Color Box"=0}, {"Mean"=0.0, " St Dev."=0.0, "Color Box"=0}, {"Mean"=0.0, " St Dev."=0.0, "Color Box"=0}, {"Mean"=0.0, " St Dev."=0.0, "Color Box"=0}, {"Mean"=0.0, " St Dev."=0.0, "Color Box"=0}, {"Mean"=0.0, " St Dev."=0.0, "Color Box"=0}, {"Mean"=0.0, " St Dev."=0.0, "Color Box"=0}, {"Mean"=0.0, " St Dev."=0.0, "Color Box"=0}, {"Mean"=0.0, " St Dev."=0.0, "Color Box"=0}, {"Mean"=0.0, " St Dev."=0.0, "Color Box"=0}, {"Mean"=0.0, " St Dev."=0.0, "Color Box"=0}, {"Mean"=0.0, " St Dev."=0.0, "Color Box"=0}, {"Mean"=0.0, " St Dev."=0.0, "Color Box"=0}, {"Mean"=0.0, " St Dev."=0.0, "Color Box"=0}, {"Mean"=0.0, " St Dev."=0.0, "Color Box"=0}, {"Mean"=0.0, " St Dev."=0.0, "Color Box"=0}, {"Mean"=0.0, " St Dev."=0.0, "Color Box"=0}, {"Mean"=0.0, " St Dev."=0.0, "Color Box"=0}, {"Mean"=0.0, " St Dev."=0.0, "Color Box"=0}, {"Mean"=0.0, " St Dev."=0.0, "Color Box"=0}, {"Mean"=0.0, " St Dev."=0.0, "Color Box"=0}, {"Mean"=0.0, " St Dev."=0.0, "Color Box"=0}, {"Mean"=0.0, " St Dev."=0.0, "Color Box"=0}, {"Mean"=0.0, " St Dev."=0.0, "Color Box"=0}, {"Mean"=0.0, " St Dev."=0.0, "Color Box"=0}, {"Mean"=0.0, " St Dev."=0.0, "Color Box"=0}, {"Mean"=0.0, " St Dev."=0.0, "Color Box"=0}, {"Mean"=0.0, " St Dev."=0.0, "Color Box"=0}, {"Mean"=0.0, " St Dev."=0.0, "Color Box"=0}, {"Mean"=0.0, " St Dev."=0.0, "Color Box"=0}, {"Mean"=0.0, " St Dev."=0.0, "Color Box"=0}, {"Mean"=0.0, " St Dev."=0.0, "Color Box"=0}, {"Mean"=0.0, " St Dev."=0.0, "Color Box"=0}, {"Mean"=0.0, " St Dev."=0.0, "Color Box"=0}, {"Mean"=0.0, " St Dev."=0.0, "Color Box"=0}, {"Mean"=0.0, " St Dev."=0.0, "Color Box"=0}, {"Mean"=0.0, " St Dev."=0.0, "Color Box"=0}, {"Mean"=0.0, " St Dev."=0.0, "Color Box"=0}, {"Mean"=0.0, " St Dev."=0.0, "Color Box"=0}, {"Mean"=0.0, " St Dev."=0.0, "Color Box"=0}, {"Mean"=0.0, " St Dev."=0.0, "Color Box"=0}, {"Mean"=0.0, " St Dev."=0.0, "Color Box"=0}, {"Mean"=0.0, " St Dev."=0.0, "Color Box"=0}, {"Mean"=0.0, " St Dev."=0.0, "Color Box"=0}, {"Mean"=0.0, " St Dev."=0.0, "Color Box"=0}, {"Mean"=0.0, " St Dev."=0.0, "Color Box"=0}, {"Mean"=0.0, " St Dev."=0.0, "Color Box"=0}, {"Mean"=0.0, " St Dev."=0.0, "Color Box"=0}, {"Mean"=0.0, " St Dev."=0.0, "Color Box"=0}, {"Mean"=0.0, " St Dev."=0.0, "Color Box"=0}, {"Mean"=0.0, " St Dev."=0.0, "Color Box"=0}, {"Mean"=0.0, " St Dev."=0.0, "Color Box"=0}, {"Mean"=0.0, " St Dev."=0.0, "Color Box"=0}, {"Mean"=0.0, " St Dev."=0.0, "Color Box"=0}, {"Mean"=0.0, " St Dev."=0.0, "Color Box"=0}, {"Mean"=0.0, " St Dev."=0.0, "Color Box"=0}, {"Mean"=0.0, " St Dev."=0.0, "Color Box"=0}, {"Mean"=0.0, " St Dev."=0.0, "Color Box"=0}, {"Mean"=0.0, " St Dev."=0.0, "Color Box"=0}, {"Mean"=0.0, " St Dev."=0.0, "Color Box"=0}, {"Mean"=0.0, " St Dev."=0.0, "Color Box"=0}, {"Mean"=0.0, " St Dev."=0.0, "Color Box"=0}, {"Mean"=0.0, " St Dev."=0.0, "Color Box"=0}, {"Mean"=0.0, " St Dev."=0.0, "Color Box"=0}, {"Mean"=0.0, " St Dev."=0.0, "Color Box"=0}, {"Mean"=0.0, " St Dev."=0.0, "Color Box"=0}, {"Mean"=0.0, " St Dev."=0.0, "Color Box"=0}, {"Mean"=0.0, " St Dev."=0.0, "Color Box"=0}, {"Mean"=0.0, " St Dev."=0.0, "Color Box"=0}, {"Mean"=0.0, " St Dev."=0.0, "Color Box"=0}, {"Mean"=0.0, " St Dev."=0.0, "Color Box"=0}, {"Mean"=0.0, " St Dev."=0.0, "Color Box"=0}, {"Mean"=0.0, " St Dev."=0.0, "Color Box"=0}, {"Mean"=0.0, " St Dev."=0.0, "Color Box"=0}, {"Mean"=0.0, " St Dev."=0.0, "Color Box"=0}, {"Mean"=0.0, " St Dev."=0.0, "Color Box"=0}, {"Mean"=0.0, " St Dev."=0.0, "Color Box"=0}, {"Mean"=0.0, " St Dev."=0.0, "Color Box"=0}, {"Mean"=0.0, " St Dev."=0.0, "Color Box"=0}, {"Mean"=0.0, " St Dev."=0.0, "Color Box"=0}, {"Mean"=0.0, " St Dev."=0.0, "Color Box"=0}, {"Mean"=0.0, " St Dev."=0.0, "Color Box"=0}, {"Mean"=0.0, " St Dev."=0.0, "Color Box"=0}, {"Mean"=0.0, " St Dev."=0.0, "Color Box"=0}, {"Mean"=0.0, " St Dev."=0.0, "Color Box"=0}, {"Mean"=0.0, " St Dev."=0.0, "Color Box"=0}, {"Mean"=0.0, " St Dev."=0.0, "Color Box"=0}, {"Mean"=0.0, " St Dev."=0.0, "Color Box"=0}, {"Mean"=0.0, " St Dev."=0.0, "Color Box"=0}, {"Mean"=0.0, " St Dev."=0.0, "Color Box"=0}, {"Mean"=0.0, " St Dev."=0.0, "Color Box"=0}, {"Mean"=0.0, " St Dev."=0.0, "Color Box"=0}, {"Mean"=0.0, " St Dev."=0.0, "Color Box"=0}, {"Mean"=0.0, " St Dev."=0.0, "Color Box"=0}, {"Mean"=0.0, " St Dev."=0.0, "Color Box"=0}, {"Mean"=0.0, " St Dev."=0.0, "Color Box"=0}, {"Mean"=0.0, " St Dev."=0.0, "Color Box"=0}, {"Mean"=0.0, " St Dev."=0.0, "Color Box"=0}, {"Mean"=0.0, " St Dev."=0.0, "Color Box"=0}, {"Mean"=0.0, " St Dev."=0.0, "Color Box"=0}, {"Mean"=0.0, " St Dev."=0.0, "Color Box"=0}]  # Test Data Array
        w137 = T8 {"Current VI Reference"=refnum, "Close Panel on Exit?"=FALSE}  # Core
        # "MW100 References"
        # "EQUIP VISA References"
        # "do not delete - used by framework"
        # "Data names and types of shift register data are defined by this bundle."
        # "Initialize the shift-register data, here.\n(data names are defined by what you wire into the bundle function)"
        n45 = call "Semiphore-Create-Local.vi"("Semiphore"="Semiphore", "error in (no error)"=w127) -> ("semaphore"=w129:T3, "error out"=w126:errorcluster)  [unwired: 15 in, 1 out]
        n46 = Unbundle("Equipment") -> ("MW100"=w134:refnum<visa-resource-name>, "AG34970"=w133:refnum<visa-resource-name>, "Chamber"=w132:refnum<visa-resource-name>)  [unwired: 1 out]
        n47 = Bundle By Name(cluster="Equipment", "COM Port"="COM Port", "MW100"=w134, "AG34970"=w133, "Chamber"=w132) -> (w130:T4)
        n48 = call "HEWH InitializeEquipmet.vi"("Semiphore"=w129, "Error In"=w126, "Equipment"=w130) -> ("Error Out"=w124:errorcluster, "Equipment Out"=w128:T4)  [unwired: 5 in, 2 out]
        n49 = property class="Instr"(reference="COM Port", error in=w124) -> (error out=w122:errorcluster, "General Settings:Timeout Value"=w123:u32)  [unwired: 1 out]
        "Com Port Timeout Value" <- w123
        n50 = Bundle("Core"=w137, "Num Samples"="Num Samples", "Equipment Out"=w128, "semaphore"=w129, "Timeout"=w123, "Test Data Array"=w121) -> (w138:T7)  [unwired: 1 in]
        n51 = call <vilib>:"Add State(s) to Queue__jki_lib_state_machine.vi"("State(s) in (\"\")"=w140) -> ("States Out"=w139:string)  [unwired: 14 in]
      }
      frame #8 {
        # "Reset Timeout to Initial Value"
        # "Cleanup any data and references, here.\n(this is called automatically, by the Macro: Exit)"
        n52 = Unbundle By Name(w145) -> ("Core.Current VI Reference"=w147:refnum<vi>, "semaphore"=w144:T3, "Equipment Out"=w143:T4)  [unwired: 2 out]
        n53 = call "HEWH CloseEquipmet.vi"("Semiphore"=w144, "Error In"=w141, "Equipment"=w143) -> ("Error Out"=w142:errorcluster)  [unwired: 8 in]
        n54 = Close Reference(reference=w147, error in (no error)=w142) -> (error out=w146:errorcluster)
        n55 = call <vilib>:"Add State(s) to Queue__jki_lib_state_machine.vi"("State(s) in (\"\")"=w149) -> ("States Out"=w148:string)  [unwired: 14 in]
      }
      frame #9 {
        # "Do not put any code in this frame.\n(It is a separator no-op. You can make a copy of this frame to create a new UI frame)"
        n56 = call <vilib>:"Add State(s) to Queue__jki_lib_state_machine.vi"("State(s) in (\"\")"=w153) -> ("States Out"=w152:string)  [unwired: 14 in]
      }
      frame #10 {
        w158 = T1 {"Mean"=99.0, " St Dev."=99.0, "Color Box"=16318226} ("Sensor")
        # "Initialize the User Interface, here.\n(this is called automatically, by the Macro: Init)"
        n57 = stacked-sequence {
          tunnel: "Panel 1" -> [w166 w179]
          tunnel: w158 -> [w165 w178]
          tunnel: [w164 _] -> w157
          tunnel: "Panel 2" -> [_ _]
          tunnel: "Panel 3" -> [_ _]
          tunnel: [_ w176] -> w154
          frame #0 {
            n58 = for {
              tunnel: w166 -> [w169] mode=indexing
              tunnel: w165 -> [w168]
              tunnel: [w167] -> w164 mode=indexing
              n59 = for {
                tunnel: w169 -> [w175] mode=indexing
                tunnel: w168 -> [w174]
                tunnel: [w170] -> w167 mode=indexing
                n60 = Unbundle(w174) -> ("Mean"=w173:dbl, "St Dev."=w172:dbl, "Color Box"=w171:u32)
                n61 = Bundle By Name(cluster=w175, "Mean"=w173, "St Dev."=w172, "Color Box"=w171) -> (w170:T1)
              }
            }
          }
          frame #1 {
            n62 = for {
              N: 3 -> [_]
              tunnel: w179 -> [_] mode=indexing
              tunnel: w178 -> [w180]
              tunnel: [w180] -> w176 mode=indexing
            }
          }
        }
        "Temperatures" <- w154
        "Pressures" <- w154
        n63 = local write "Panel 1"(w157) -> ()
        n64 = local write "Panel 2"(w157) -> ()
        n65 = local write "Panel 3"(w157) -> ()
        n66 = call <vilib>:"Add State(s) to Queue__jki_lib_state_machine.vi"("State(s) in (\"\")"=w163) -> ("States Out"=w162:string)  [unwired: 14 in]
        "Power" <- w158
        "Tc Down" <- w158
      }
      frame #11 {
        # "Argument"
        # "Set and Unset Cursor Busy.\n(Usage: \"UI: Cursor Set >> Busy|Idle\")"
        n67 = case shown="\"Idle\", Default" w181 {
          tunnel: w183 -> [w188 w190]
          tunnel: [w187 w189] -> w182
          frame #0 {
            n68 = call <vilib>:"Unset Busy.vi"("error in (no error)"=w188) -> ("error out"=w187:errorcluster)  [unwired: 10 in]
          }
          frame #1 {
            n69 = call <vilib>:"Set Busy.vi"("error in (no error)"=w190) -> ("error out"=w189:errorcluster)  [unwired: 9 in, 1 out]
          }
        }
        n70 = call <vilib>:"Add State(s) to Queue__jki_lib_state_machine.vi"("State(s) in (\"\")"=w186) -> ("States Out"=w185:string)  [unwired: 14 in]
      }
      frame #12 {
        # "Argument"
        # "Set Front Panel Open or Closed\n(Usage: \"UI: Front Panel State >> Open|Close\")"
        n71 = Unbundle By Name(w193) -> ("Core.Current VI Reference"=w192:refnum<vi>)
        n72 = case shown="\"Close\"" w191 {
          tunnel: w195 -> [w201 w214]
          tunnel: [w203 w215] -> w194
          tunnel: w192 -> [w202 w212]
          frame #0 {
            n73 = property class="VI"(reference=w202, error in=w201) -> (reference out=w199:refnum<vi>, error out=w200:errorcluster, "Front Panel.Open"=w198:bool)
            n74 = case shown="False" w198 {
              tunnel: [w206 w209] -> w203
              tunnel: w200 -> [w205 w209]
              tunnel: w199 -> [w204 _]
              frame #0 {
                n75 = invoke class="VI" method="FP.Open"(reference=w204, error in=w205, "Activate"=TRUE, "State"=T6."Standard") -> (error out=w206:errorcluster)  [unwired: 1 in, 4 out]
              }
              frame #1 {
              }
            }
          }
          frame #1 {
            n76 = property class="VI"(reference=w212, error in=w214) -> (reference out=w211:refnum<vi>, error out=w213:errorcluster, "Front Panel.Open"=w210:bool)
            n77 = case shown="True" w210 {
              tunnel: [w216 w219] -> w215
              tunnel: w213 -> [w216 w218]
              tunnel: w211 -> [_ w217]
              frame #0 {
              }
              frame #1 {
                n78 = invoke class="VI" method="FP.Close"(reference=w217, error in=w218) -> (error out=w219:errorcluster)  [unwired: 1 in, 2 out]
              }
            }
          }
        }
        n79 = call <vilib>:"Add State(s) to Queue__jki_lib_state_machine.vi"("State(s) in (\"\")"=w197) -> ("States Out"=w196:string)  [unwired: 14 in]
      }
      frame #13 {
        # "Do not put any code in this frame.\n(It is a separator no-op. You can make a copy of this frame to create a new Macro frame)"
        n80 = call <vilib>:"Add State(s) to Queue__jki_lib_state_machine.vi"("State(s) in (\"\")"=w223) -> ("States Out"=w222:string)  [unwired: 14 in]
      }
      frame #14 {
        w224 = "Data: Initialize\nInitialize Core Data\nUI: Initialize\nUI: Front Panel State >> Open"  # Data: Initialize Initialize Core Data UI: Initialize UI: Front Panel State >> Open
        # "Initialization Macro\n(This is called once, when the VI starts)"
        n81 = call <vilib>:"Add State(s) to Queue__jki_lib_state_machine.vi"("State(s) in Front (\"\")"=w224, "State(s) in (\"\")"=w228) -> ("States Out"=w227:string)  [unwired: 13 in]
      }
      frame #15 {
        # "Exit Macro\n(This is called once, when the VI exits)"
        n82 = Unbundle By Name(w235) -> ("Core.Close Panel on Exit?"=w234:bool)
        n83 = Select(t="UI: Front Panel State >> Close", s=w234, f="") -> (s? t:f=w231:string)
        n84 = call <vilib>:"Add State(s) to Queue__jki_lib_state_machine.vi"("State(s) in (\"\")"=w231, "State(s) at Back (\"\")"="Data: Cleanup\nExit") -> ("States Out"=w229:string)  [unwired: 13 in]
        n85 = call <vilib>:"Add State(s) to Queue__jki_lib_state_machine.vi"("State(s) in Front (\"\")"=w229, "State(s) in (\"\")"=w238) -> ("States Out"=w237:string)  [unwired: 13 in]
      }
      frame #16 {
        # "Template Separator\n(You can make a copy of, or modify, this frame)"
        n86 = call <vilib>:"Add State(s) to Queue__jki_lib_state_machine.vi"("State(s) in (\"\")"=w242) -> ("States Out"=w241:string)  [unwired: 14 in]
      }
      frame #17 {
        # "Your code here.\n(You can make a copy of, or modify, this frame)"
        n87 = call <vilib>:"Add State(s) to Queue__jki_lib_state_machine.vi"("State(s) in (\"\")"=w247, "State(s) at Back (\"\")"="TestDAQ: Gather\nTestDAQ: Sort\nTestDAQ: Verify" ("State(s) at Back (\"\")")) -> ("States Out"=w246:string)  [unwired: 13 in]
      }
      frame #18 {
        # "Your code here.\n(You can make a copy of, or modify, this frame)"
        n88 = Unbundle By Name(w265) -> ("Equipment Out.COM Port"=w254:refnum<visa-resource-name>, "Num Samples"=w258:i32)
        n89 = property class="Instr"(reference=w254, error in=w255) -> (reference out=w250:refnum<visa-resource-name>, error out=w251:errorcluster, "General Settings:Timeout Value"=w253:u32)
        n90 = property class="Instr"(reference=w250, error in=w251, "General Settings:Timeout Value"=u32 500) -> (error out=w249:errorcluster)  [unwired: 1 out]
        n91 = for {
          N: w258 -> [_]
          tunnel: w254 -> [w272]
          tunnel: w249 -> [w268]
          shift-right: [w271] -> w256
          shift-left: i16 0 -> [w270]
          tunnel: [w268] -> w248
          i -> [w269]
          w276 = "This is a test 12345678910."
          n92 = local write "Data Sample"(w269) -> ()
          n93 = VISA Write(VISA resource name=w272, write buffer=w276, error in (no error)=w268) -> (VISA resource name out=w279:refnum<visa-resource-name>, error out=w280:errorcluster)  [unwired: 1 out]
          n94 = String Length(string=w276) -> (length=w275:i32)
          n95 = VISA Read(VISA resource name=w279, byte count=w275, error in (no error)=w280) -> (read buffer=w278:string, error out=→"serial error out":errorcluster)  [unwired: 2 out]
          n96 = Equal?(x=w276, y=w278) -> (x = y?=w273:bool)
          n97 = Boolean To (0,1)(Boolean=w273) -> (0, 1=w274:i16)
          n98 = Add(x=w270, y=w274) -> (x+y=w271:i16)
        }
        n99 = Equal?(x=w258, y=w256) -> (x = y?=w257:bool)
        n100 = Select(t=u32 5373696 ("Color Box"), s=w257, f=u32 16711722 ("Color Box")) -> (s? t:f=w259:u32)
        n101 = Bundle By Name(cluster=cluster{"Num OK":i16, "Color Box":u32} {"Num OK"=0, "Color Box"=5373696} ("Sensor"), "Num OK"=w256, "Color Box"=w259) -> (→"Serial Loopback":cluster{"Num OK":i16, "Color Box":u32})
        n102 = property class="Instr"(reference=w254, error in=w248, "General Settings:Timeout Value"=w253) -> ()  [unwired: 2 out]
        n103 = call <vilib>:"Add State(s) to Queue__jki_lib_state_machine.vi"("State(s) in (\"\")"=w267) -> ("States Out"=w266:string)  [unwired: 14 in]
      }
      frame #19 {
        # "Template Separator\n(You can make a copy of, or modify, this frame)"
        n104 = call <vilib>:"Add State(s) to Queue__jki_lib_state_machine.vi"("State(s) in (\"\")"=w284) -> ("States Out"=w283:string)  [unwired: 14 in]
      }
      frame #20 {
        # "Template Separator\n(You can make a copy of, or modify, this frame)"
        n105 = Unbundle By Name(w289) -> ("Equipment Out"=w292:T4, "semaphore"=w290:T3, "Num Samples"=w291:i32)
        n106 = for {
          N: w291 -> [_]
          tunnel: w290 -> [w313]
          tunnel: [w316] -> w286 mode=indexing
          shift-right: [w314] -> w293
          shift-left: w294 -> [w306]
          tunnel: w292 -> [w303]
          i -> [w315]
          n107 = control-ref of="Local Tank Display"() -> (w305:refnum<vi>)
          n108 = call "Agilent_Get_ScanList.vi"() -> ("Scanlist"=w307:string)  [unwired: 11 in]
          n109 = call "Gather Test Data - Heatup Test new.vi"("Agilent Scan List"=w307, "Semiphore"=w313, "Equipment"=w303, "Tank Display Ref"=w305, "Agilent?"=TRUE ("No Serial?"), "error in (no error)"=w306, "Serial Data In"="0:0:0 UE 24 LE 24 COMP 0 FAN1 0 FAN2 0 SP:0 0 0 0 0 0 C030" ("trimmed string"), "Agilent Label Array"=string[] ["TC Evap1 - IN", "TC Evap2", "TC Evap3", "TC Evap4", "TC Evap5 - OUT", "TC Xtra 1", "TC Xtra 2", "TC Xtra 3", "TC Xtra 4", "TC Dry/W bulb 1", "TC Dry/W bulb 2", "TC Dry/W bulb 3", "TC Dry/W bulb 4", "TC Tsuct", "TC Tdis", "TC Tret", "TC Controls 1", "TC Controls 2", "TC Controls 3", "TC Controls 4", "TC Controls 5", "TC Shadow T1", "TC Shadow T2", "TC Shadow T3", "TC Shadow T4", "TC Shadow T5", "TC Shadow T6", "TC Xtra 5", "TC Xtra 6", "TC Xtra 7", "TC Xtra 8", "TC Xtra 9", "TC Cond1 - IN", "TC Cond2", "TC Cond3", "TC Cond4", "TC Cond5", "TC Cond6", "TC Cond7", "TC Cond8", "TC Cond9", "TC Cond10", "TC Cond11", "TC Cond12 - OUT", "NC", "NC", "NC", "NC"] ("output array")) -> ("Output Data"=w309:string[][], "error out"=w314:errorcluster)  [unwired: 2 in, 4 out]
          n110 = Array Size(array=w309) -> (size(s)=w312:i32[])
          n111 = Array Max & Min(array=w312) -> (max value=w311:i32)  [unwired: 3 out]
          n112 = Index Array(array=w309, index (row)=1 ("index")) -> (element=w308:string[])  [unwired: 1 in]
          n113 = Reshape Array(w308, w311) -> (w317:string[])
          n114 = Fract/Exp String To Number(string=w317) -> (number=w316:dbl[])  [unwired: 3 in, 1 out]
          "Data Sample" <- w315
        }
        n115 = Transpose 2D Array(2D array=w286) -> (transposed array=w285:dbl[][])
        n116 = for {
          tunnel: w285 -> [w301] mode=indexing
          tunnel: [w298] -> w288 mode=indexing
          n117 = call <vilib>:"Std Deviation and Variance.vi"("X"=w301) -> ("mean"=w300:dbl, "standard deviation"=w299:dbl)  [unwired: 1 in, 1 out]
          n118 = Bundle By Name(cluster=T1 {"Mean"=0.0, " St Dev."=0.0, "Color Box"=5373696} ("Sensor"), "Mean"=w300, "St Dev."=w299) -> (w298:T1)
        }
        n119 = Bundle By Name(cluster=w289, "Test Data Array"=w288) -> (w287:T7)
        n120 = call <vilib>:"Add State(s) to Queue__jki_lib_state_machine.vi"("State(s) in (\"\")"=w296) -> ("States Out"=w295:string)  [unwired: 14 in]
      }
      frame #21 {
        # "Template Separator\n(You can make a copy of, or modify, this frame)"
        n121 = Unbundle By Name(w320) -> ("Test Data Array"=w319:T1[])
        n122 = stacked-sequence {
          tunnel: w319 -> [w332 w354 w375 w395]
          frame #0 {
            n123 = local read "Panel 1"() -> (w324:T1[][])
            n124 = Array Subset(array=w332, index=39, length=2) -> (w329:T1[])
            n125 = Array Subset(array=w332, index=23, length=6) -> (w328:T1[])
            n126 = Array Subset(array=w332, index=22, length=1) -> (w331:T1[])
            n127 = Array Subset(array=w332, index=30, length=3) -> (w330:T1[])
            n128 = Array Subset(array=w332, index=41, length=6) -> (w326:T1[])
            n129 = Replace Array Subset(array=w324, new element=w328, index (row)=0) -> (w345:T1[][])  [unwired: 1 in]
            n130 = Build Array (concatenate)(w331, w330, w329) -> (w327:T1[])
            n131 = Replace Array Subset(array=w345, new element=w327, index (row)=1) -> (w343:T1[][])  [unwired: 1 in]
            n132 = Replace Array Subset(array=w343, new element=w326, index (row)=2) -> (w325:T1[][])  [unwired: 1 in]
            n133 = local write "Panel 1"(w325) -> ()
          }
          frame #1 {
            n134 = local read "Panel 2"() -> (w348:T1[][])
            n135 = Array Subset(array=w354, index=48, length=6) -> (w357:T1[])
            n136 = Array Subset(array=w354, index=54, length=6) -> (w353:T1[])
            n137 = Replace Array Subset(array=w348, new element=w357, index (row)=0) -> (w362:T1[][])  [unwired: 1 in]
            n138 = Array Subset(array=w354, index=60, length=6) -> (w352:T1[])
            n139 = Replace Array Subset(array=w362, new element=w353, index (row)=1) -> (w360:T1[][])  [unwired: 1 in]
            n140 = Replace Array Subset(array=w360, new element=w352, index (row)=2) -> (w351:T1[][])  [unwired: 1 in]
            n141 = local write "Panel 2"(w351) -> ()
          }
          frame #2 {
            (unwired) 6 ("length")
            n142 = local read "Panel 3"() -> (w365:T1[][])
            n143 = Array Subset(array=w375, index=71, length=6) -> (w370:T1[])
            n144 = Array Subset(array=w375, index=77) -> (w369:T1[])  [unwired: 1 in]
            n145 = Array Subset(array=w375, index=47, length=1) -> (w372:T1[])
            n146 = Array Subset(array=w375, index=66, length=5) -> (w371:T1[])
            n147 = Replace Array Subset(array=w365, new element=w370, index (row)=0) -> (w366:T1[][])  [unwired: 1 in]
            n148 = Build Array (concatenate)(w372, w371) -> (w368:T1[])
            n149 = Replace Array Subset(array=w366, new element=w369, index (row)=1) -> (w381:T1[][])  [unwired: 1 in]
            n150 = Replace Array Subset(array=w381, new element=w368, index (row)=2) -> (w367:T1[][])  [unwired: 1 in]
            n151 = local write "Panel 3"(w367) -> ()
          }
          frame #3 {
            # "Temperatures"
            # "Pressures"
            n152 = Index Array(array=w395, index #1=35 ("index"), index #2=33 ("index"), index #3=34 ("length")) -> (element #1=w388:T1, element #2=w387:T1, element #3=w386:T1)
            n153 = Array Subset(array=w395, index=17, length=3) -> (w392:T1[])
            n154 = Index Array(array=w395, index=29) -> (element=w394:T1)
            n155 = Index Array(array=w395, index=15) -> (element=w393:T1)
            n156 = Build Array(w388, w387, w386) -> (w385:T1[])
            n157 = local write "Pressures"(w392) -> ()
            n158 = local write "Tc Down"(w394) -> ()
            n159 = local write "Temperatures"(w385) -> ()
            n160 = local write "Power"(w393) -> ()
          }
        }
        n161 = call <vilib>:"Add State(s) to Queue__jki_lib_state_machine.vi"("State(s) in (\"\")"=w323) -> ("States Out"=w322:string)  [unwired: 14 in]
      }
      frame #22 {
        # "Template Separator\n(You can make a copy of, or modify, this frame)"
        n162 = local read "Temperatures"() -> (w400:T1[])
        n163 = local read "Pressures"() -> (w401:T1[])
        n164 = local read "Panel 3"() -> (w402:T1[][])
        n165 = local read "Panel 1"() -> (w404:T1[][])
        n166 = local read "Panel 2"() -> (w403:T1[][])
        n167 = stacked-sequence {
          tunnel: w403 -> [_ w427 _ _ _]
          tunnel: w404 -> [w409 _ _ _ _]
          tunnel: w402 -> [_ _ w443 _ _]
          tunnel: w401 -> [_ _ _ w461 _]
          tunnel: w400 -> [_ _ _ _ w476]
          frame #0 {
            n168 = for {
              tunnel: [w412] -> w410 mode=indexing
              tunnel: w409 -> [w411] mode=indexing
              n169 = for {
                tunnel: [w420] -> w412 mode=indexing
                tunnel: w411 -> [w417] mode=indexing
                n170 = Unbundle By Name(w417) -> ("Mean"=w414:dbl, "St Dev."=w421:dbl)
                n171 = In Range and Coerce(upper limit="TC Max OK Val", x=w414, lower limit="TC Min OK Val") -> (In Range?=w413:bool)  [unwired: 1 out]
                n172 = Less?(x=w421, y="StDev Thresh") -> (x < y?=w419:bool)
                n173 = And(x=w419, y=w413) -> (x .and. y?=w418:bool)
                n174 = Select(t=u32 5373696 ("Color Box"), s=w418, f=u32 16711680 ("Color Box")) -> (s? t:f=w422:u32)
                n175 = Bundle By Name(cluster=w417, "Mean"=w414, "St Dev."=w421, "Color Box"=w422) -> (w420:T1)
              }
            }
            n176 = local write "Panel 1"(w410) -> ()
          }
          frame #1 {
            n177 = for {
              tunnel: w427 -> [w429] mode=indexing
              tunnel: [w428] -> w426 mode=indexing
              n178 = for {
                tunnel: w429 -> [w442] mode=indexing
                tunnel: [w437] -> w428 mode=indexing
                n179 = local read "StDev Thresh"() -> (w434:dbl)
                n180 = local read "TC Min OK Val"() -> (w431:dbl)
                n181 = local read "TC Max OK Val"() -> (w430:dbl)
                n182 = Unbundle By Name(w442) -> ("Mean"=w433:dbl, "St Dev."=w438:dbl)
                n183 = Less?(x=w438, y=w434) -> (x < y?=w436:bool)
                n184 = In Range and Coerce(upper limit=w430, x=w433, lower limit=w431) -> (In Range?=w432:bool)  [unwired: 1 out]
                n185 = And(x=w436, y=w432) -> (x .and. y?=w435:bool)
                n186 = Select(t=u32 5373696 ("Color Box"), s=w435, f=u32 16711680 ("Color Box")) -> (s? t:f=w439:u32)
                n187 = Bundle By Name(cluster=w442, "Mean"=w433, "St Dev."=w438, "Color Box"=w439) -> (w437:T1)
              }
            }
            n188 = local write "Panel 2"(w426) -> ()
          }
          frame #2 {
            n189 = for {
              tunnel: w443 -> [w446] mode=indexing
              tunnel: [w445] -> w444 mode=indexing
              n190 = for {
                tunnel: w446 -> [w459] mode=indexing
                tunnel: [w454] -> w445 mode=indexing
                n191 = local read "TC Min OK Val"() -> (w450:dbl)
                n192 = Unbundle By Name(w459) -> ("Mean"=w449:dbl, "St Dev."=w455:dbl)
                n193 = local read "StDev Thresh"() -> (w451:dbl)
                n194 = local read "TC Max OK Val"() -> (w448:dbl)
                n195 = Less?(x=w455, y=w451) -> (x < y?=w453:bool)
                n196 = In Range and Coerce(upper limit=w448, x=w449, lower limit=w450) -> (In Range?=w447:bool)  [unwired: 1 out]
                n197 = And(x=w453, y=w447) -> (x .and. y?=w452:bool)
                n198 = Select(t=u32 5373696 ("Color Box"), s=w452, f=u32 16711680 ("Color Box")) -> (s? t:f=w456:u32)
                n199 = Bundle By Name(cluster=w459, "Mean"=w449, "St Dev."=w455, "Color Box"=w456) -> (w454:T1)
              }
            }
            n200 = local write "Panel 3"(w444) -> ()
          }
          frame #3 {
            n201 = for {
              tunnel: w461 -> [w474] mode=indexing
              tunnel: [w469] -> w460 mode=indexing
              n202 = Unbundle By Name(w474) -> ("Mean"=w463:dbl, "St Dev."=w470:dbl)
              n203 = local read "StDev Thresh"() -> (w466:dbl)
              n204 = In Range and Coerce(upper limit="PSI Max OK", x=w463, lower limit="PSI Min OK") -> (In Range?=w462:bool)  [unwired: 1 out]
              n205 = Less?(x=w470, y=w466) -> (x < y?=w468:bool)
              n206 = And(x=w468, y=w462) -> (x .and. y?=w467:bool)
              n207 = Select(t=u32 5373696 ("Color Box"), s=w467, f=u32 16711680 ("Color Box")) -> (s? t:f=w471:u32)
              n208 = Bundle By Name(cluster=w474, "Mean"=w463, "St Dev."=w470, "Color Box"=w471) -> (w469:T1)
            }
            n209 = local write "Pressures"(w460) -> ()
          }
          frame #4 {
            n210 = for {
              tunnel: w476 -> [w489] mode=indexing
              tunnel: [w484] -> w475 mode=indexing
              n211 = Unbundle By Name(w489) -> ("Mean"=w478:dbl, "St Dev."=w485:dbl)
              n212 = local read "StDev Thresh"() -> (w481:dbl)
              n213 = In Range and Coerce(upper limit="RTD Max OK", x=w478, lower limit="RTD Min OK") -> (In Range?=w477:bool)  [unwired: 1 out]
              n214 = Less?(x=w485, y=w481) -> (x < y?=w483:bool)
              n215 = And(x=w483, y=w477) -> (x .and. y?=w482:bool)
              n216 = Select(t=u32 5373696 ("Color Box"), s=w482, f=u32 16711680 ("Color Box")) -> (s? t:f=w486:u32)
              n217 = Bundle By Name(cluster=w489, "Mean"=w478, "St Dev."=w485, "Color Box"=w486) -> (w484:T1)
            }
            n218 = local write "Temperatures"(w475) -> ()
          }
        }
        n219 = call <vilib>:"Add State(s) to Queue__jki_lib_state_machine.vi"("State(s) in (\"\")"=w408) -> ("States Out"=w407:string)  [unwired: 14 in]
      }
    }
  }
